vi "SCA-RT_old_new.vi"() -> ()   [LabVIEW 2016]
uses:
  <vilib>/Platform/TimedLoop/XDataNode/wakeup.ctl
  <vilib>/Platform/TimedLoop/XDataNode/XDNodeRunTimeDep.lvlib
  <vilib>/Platform/TimedLoop/XDataNode/nitl_modes.ctl
  <vilib>/Platform/TimedLoop/XDataNode/timing_clust.ctl
  <vilib>/Platform/TimedLoop/XDataNode/XDataNode.xnode
  <vilib>/Motion/BlockNode/FB.NIMotion.xnode
  <vilib>/Platform/TimedLoop/XDataNode/loadnilvce.vi
  controls/state control sample changer.ctl
  <vilib>/Instr/_visa.llb/VISA Configure Serial Port (Instr).vi
  <vilib>/Analysis/NI_AALBase.lvlib
  <vilib>/Analysis/baseanly.llb/Mean (DBL).vi
  controls/SCA states.ctl
  controls/Encoder bit cluster.ctl
  control vi/controls/Gate Valve Readback.ctl
  controls/Horizontal Rod states.ctl
  controls/Vertical Rod states.ctl
  <vilib>/NI_Real-Time Target Support.lvlib
  <vilib>/Motion/Express/_s/nimc.fb.straightLineMove.startStraightLineMove.axis.modeRelative.0.vi
  controls/SCA broadcast status.ctl
  controls/GP307 cluster.ctl
panel:
  out "Timeouts":T1
  out "Encoder loop error":errorcluster
  out "Convectron readback loop error":errorcluster
  out "HV Control loop error":errorcluster
  out "Rotate Wheel error":errorcluster
  out "Ion Source Vac Cluster":T2
  out "Bellows Vac Cluster":T2
  out "Start Sample Change":bool
  out "SCA-cRIO error":errorcluster
  in  "Rollover Sample":i8=54
  out "Insert Rod Status":T3
  out "Retract Rod Status":T3
  out "Sample Rod status":T4
  out "Wheel GV":T5
  out "Raw bits":bool[](array[boolean])
  out "Converted bits":bool[](array[boolean])
  out "Immersion Lens I read":dbl format="%0.2f"
  out "Immersion Lens V read":dbl format="%0.2f"
  out "SCA next state":T6
  out "Extractor I read":dbl
  out "Extractor V read":dbl
  out "Extractor V set":dbl
  out "Cathode V read":dbl
  out "Cathode I read":dbl
  out "Cathode V set":dbl
  in  "Execute Move":bool
  out "New Move":dbl
  out "Encoder Destination":dbl
  in  "Step Window Radius":i16=2
  out "In Range?":bool
  out "Window Limit 2":u32
  out "Window Limit 1":u32
  out "Encoder position":u16
  out "change sample start end":bool
  out "start sample change":bool
  in  "clear error 3":bool
  in  "clear error 2":bool
  out "set cold cathode on 2":bool
  out "Rotate Wheel":bool
  out "Venting Source":bool
  out "Pumping out Source":bool
  out "insert Retract Rod":bool
  out "retract Retract Rod":bool
  out "Open Wheel GV":bool
  out "Close Wheel GV":bool
  out "insert Insert Rod":bool
  out "retract Insert Rod":bool
  out "insert Sample Rod":bool
  out "retract Sample Rod":bool
  in  "clear error":bool
  out "action":string
  out "Vac Readback Loop error":errorcluster
  out "Sample Wheel Convectron":string
  out "Sample Rod UP sensor":bool
  out "Sample Rod DOWN sensor":bool
  out "done":bool
  out "Insert Rod IN sensor":bool
  out "Insert Rod OUT sensor":bool
  out "Retract Rod IN sensor":bool
  out "Retract Rod OUT sensor":bool
  out "Sensor loop error":errorcluster
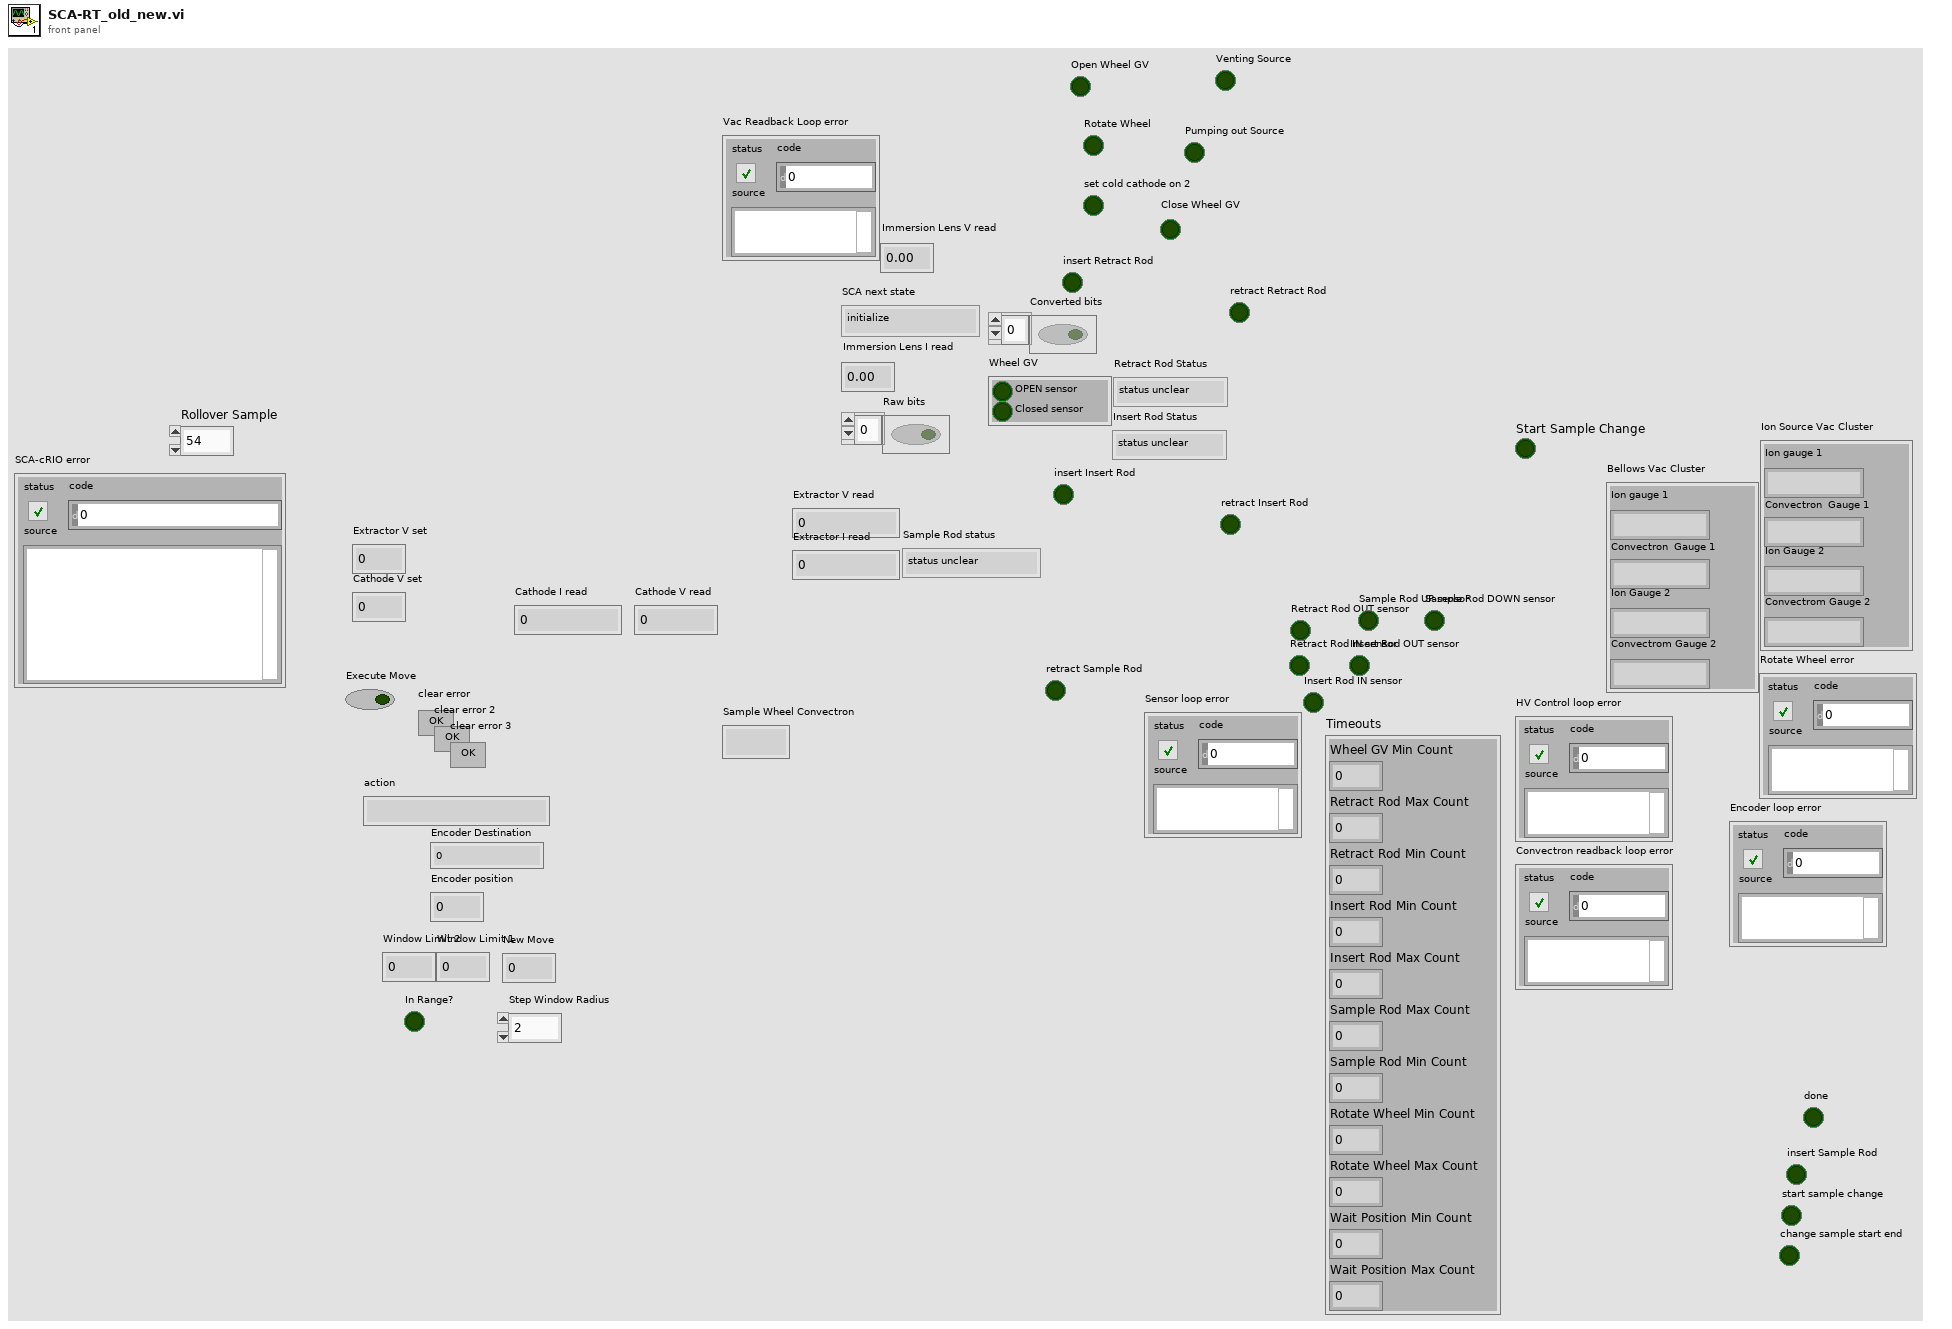
[diagram p1: front panel]
types:
  T1 = cluster{"Wheel GV Min Count":i32, "Retract Rod Max Count":u32, "Retract Rod Min Count":u32, "Insert Rod Min Count":u32, "Insert Rod Max Count":u32, "Sample Rod Max Count":u32, "Sample Rod Min Count":u32, "Rotate Wheel Min Count":u32, "Rotate Wheel Max Count":u32, "Wait Position Min Count":u32, "Wait Position Max Count":u32}
  T2 = typedef "GP307 cluster.ctl" = cluster{"Ion gauge 1":string, "Convectron  Gauge 1 ":string, "Ion Gauge 2":string, "Convectrom Gauge 2":string}
  T3 = typedef "Horizontal Rod states.ctl" = enum16{"status unclear", "rod in", "rod out"}
  T4 = typedef "Vertical Rod states.ctl" = enum16{"status unclear", "rod down", "rod up"}
  T5 = typedef "Gate Valve Readback.ctl" = cluster{"OPEN sensor":bool, "Closed sensor":bool}
  T6 = typedef "SCA states.ctl" = enum16{"initialize", "wait", "change sample start", "change sample", "check position", "rotate wheel", "sample change complete", "sample rod up", "sample rod down", "retract rod in", "retract rod out", "insert rod in", "insert rod out", "wheel GV open", "wheel GV close", "vent source", "pump source", "shutdown"}
  T7 = typedef "SCA broadcast status.ctl" = enum16{"Waiting", "Changing samples", "Sample change complete", "Failure"}
  T8 = typedef "SCA states.ctl" = enum16{"initialize", "wait", "change sample start", "change sample", "check position", "wait position", "rotate wheel", "sample change complete", "sample rod up", "sample rod down", "retract rod in", "retract rod out", "insert rod in", "insert rod out", "wheel GV open", "wheel GV close", "vent source", "pump source"}
  T9 = typedef "GV states.ctl" = enum16{"status unclear", "closed", "open"}
  T10 = typedef "XDNodeRunTimeDep.lvlib/timing_clust.ctl" = cluster{"Expected End [f-1]":u64, "Actual End [f-1]":u64, "Finished Late? [f-1]":bool, "Expected End [i-1]":u64, "Actual End [i-1]":u64, "Finished Late? [i-1]":bool, "Expected Start [i]":u64, "Actual Start [i]":u64, "Expected Start [f]":u64, "Actual Start [f]":u64, "Source Name":string, "Structure Name":string, "Period":i64, "Deadline":i64, "Offset":i64, "Start":i64, "Priority":i32, "Timeout":i32, "Mode":T11, "Wakeup Reason":T12, "Error":errorcluster, "Source Type":string, "Secondary Source Type":string, "Global End Time":u64, "Global Start Time":u64, "Frame Duration":u64, "Iteration Duration":u64, "Assigned CPU":i32, "I/O Scan Engine Mode":u32}
  T11 = typedef "XDNodeRunTimeDep.lvlib/nitl_modes.ctl" = enum32{"No Change", "Process missed periods, maintain original phase", "Discard missed periods, maintain original phase", "Process missed periods, ignore original phase", "Discard missed periods, ignore original phase"}
  T12 = typedef "XDNodeRunTimeDep.lvlib/wakeup.ctl" = enum32{"Normal", "Aborted", "Asynchronous wakeup", "Timing source error", "Timed loop error", "Timeout"}
  T13 = typedef "Encoder bit cluster.ctl" = cluster{"MSB":bool, "13th bit":bool, "12th bit":bool, "11th bit":bool, "10th bit":bool, "9th bit":bool, "8th bit":bool, "7th bit":bool, "6th bit":bool, "5th bit":bool, "4th bit":bool, "3rd bit":bool, "2nd bit":bool, "LSB":bool}
  T14 = typedef "state control sample changer.ctl" = string
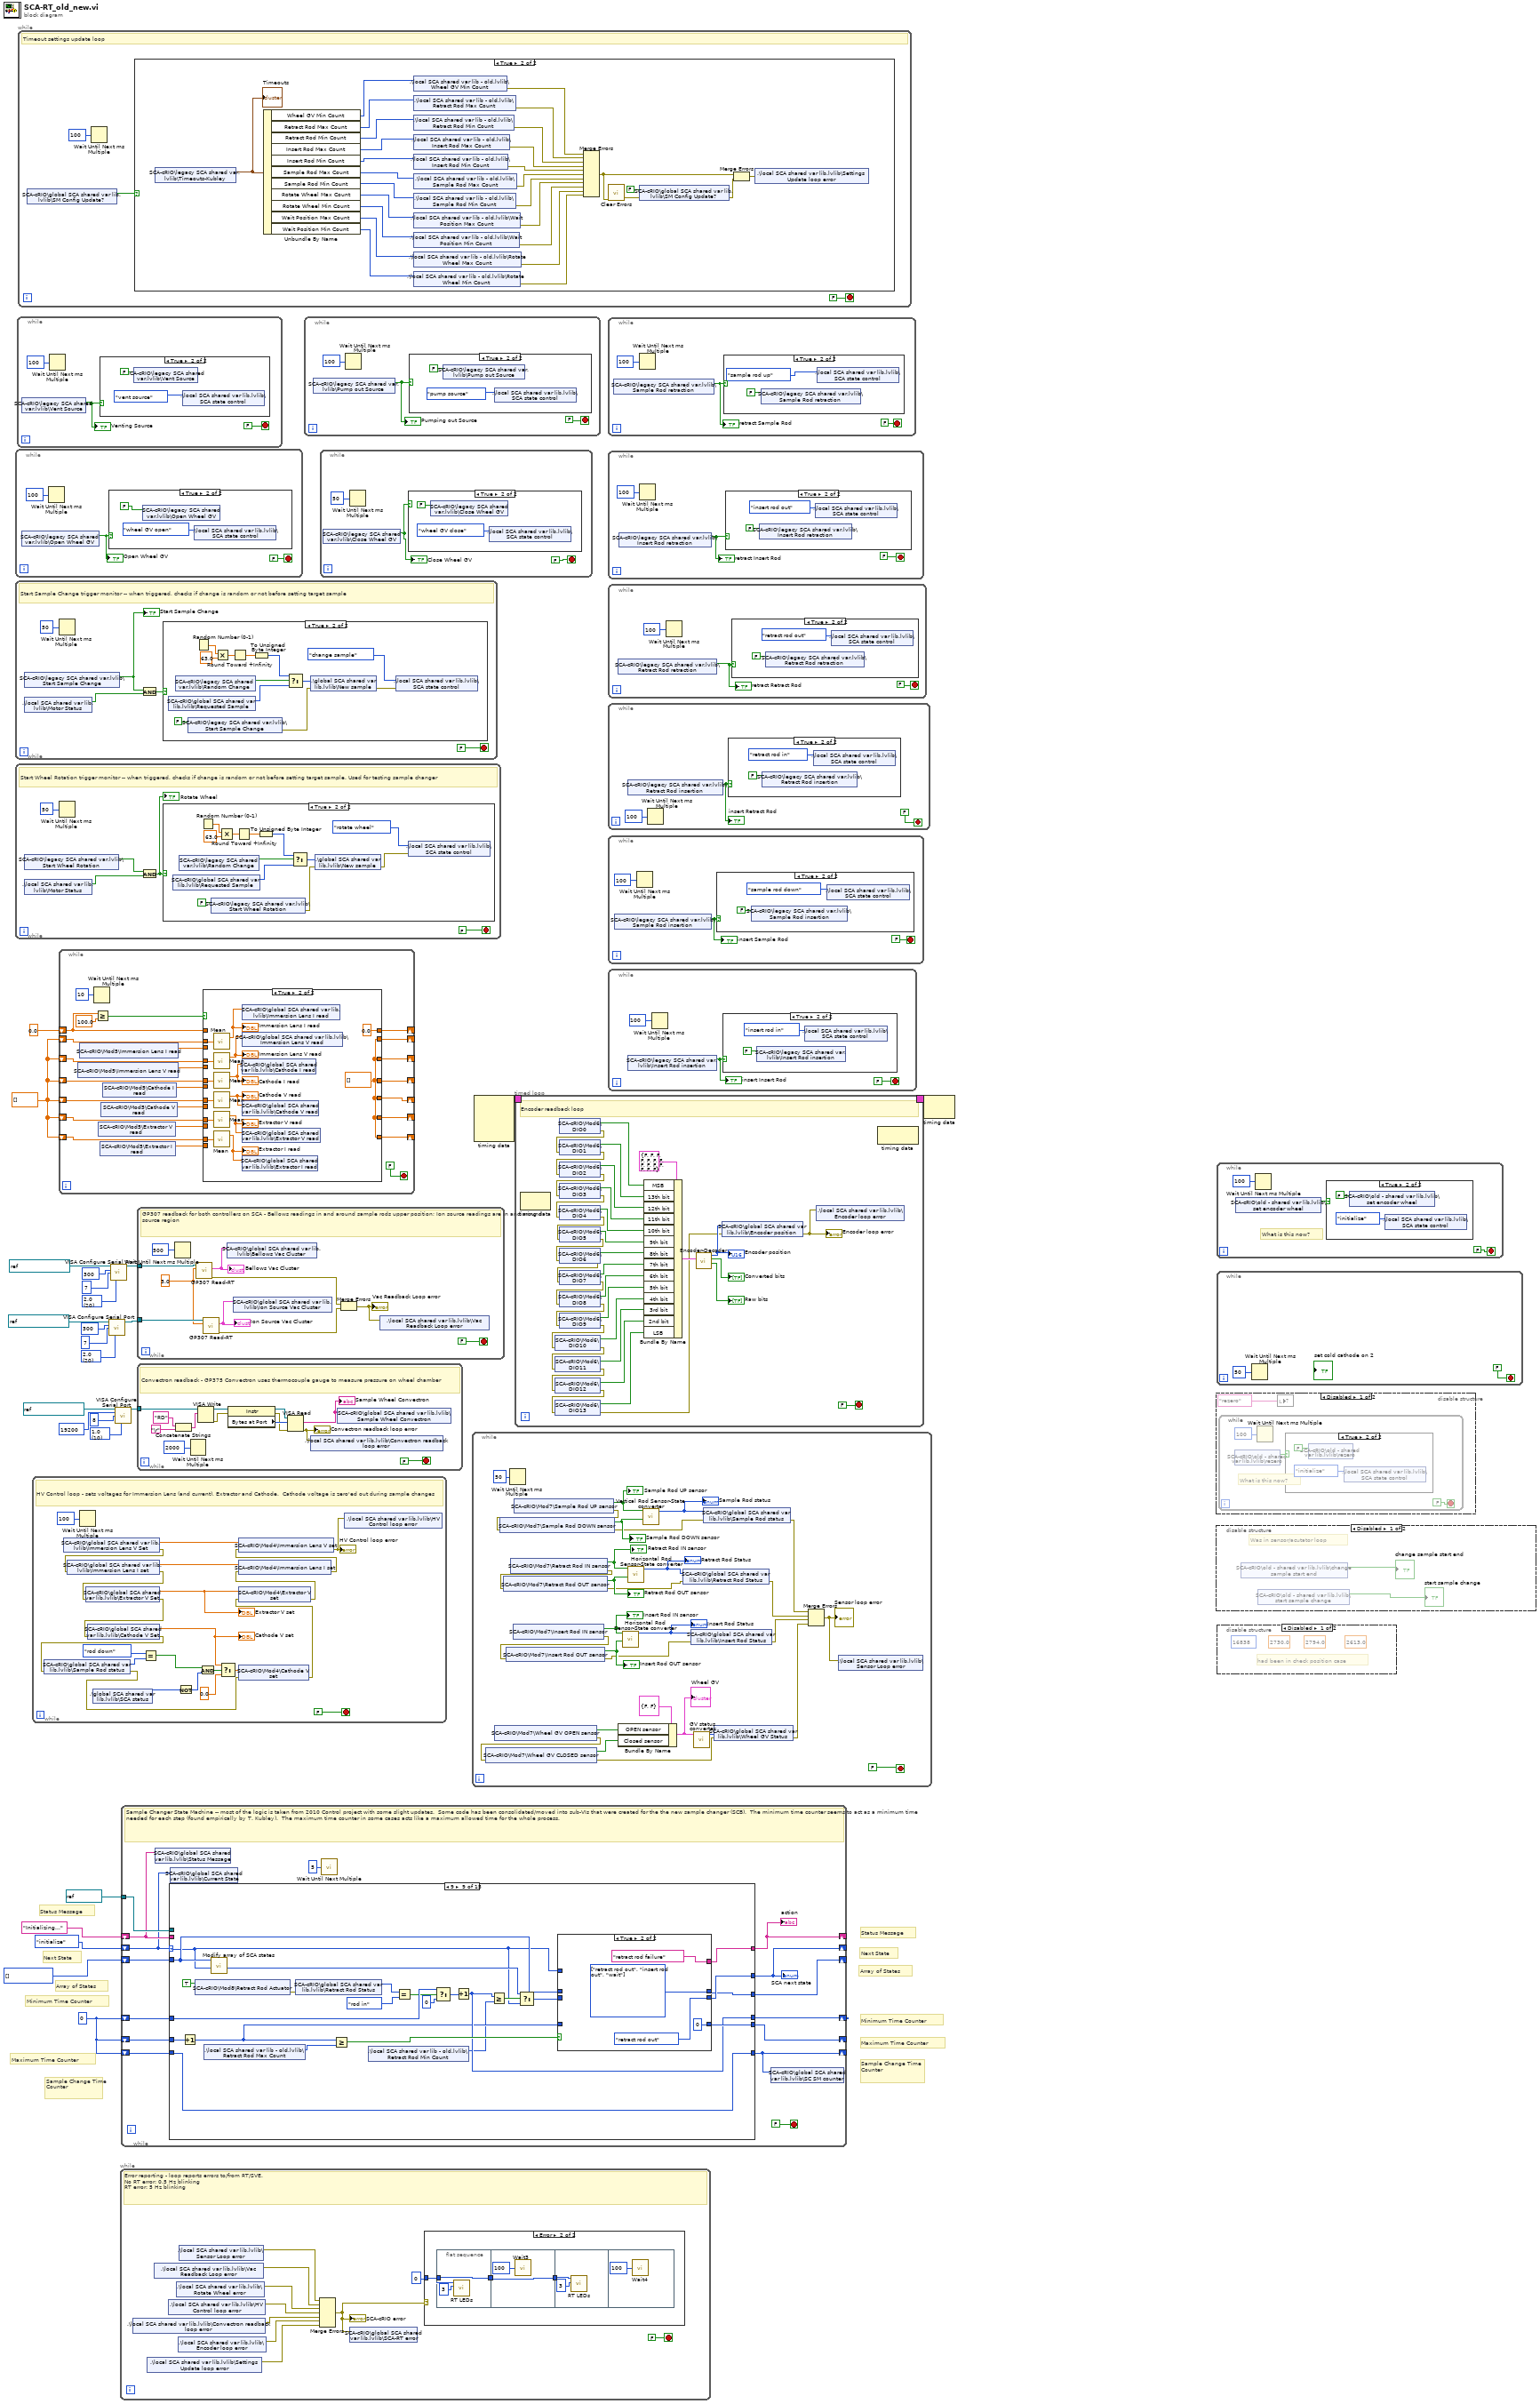
[diagram p0: block diagram]
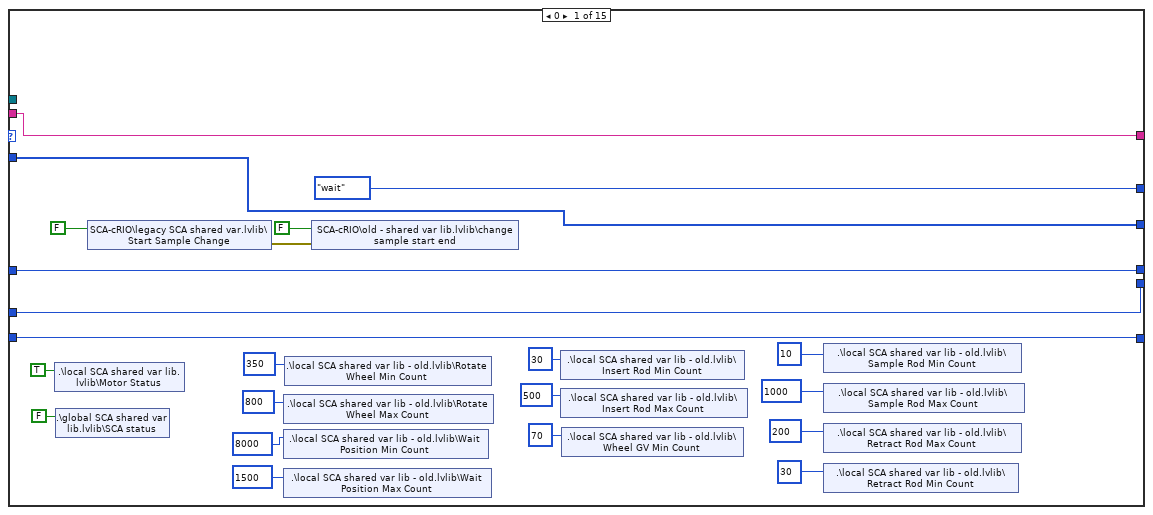
[diagram p5: hidden frame]
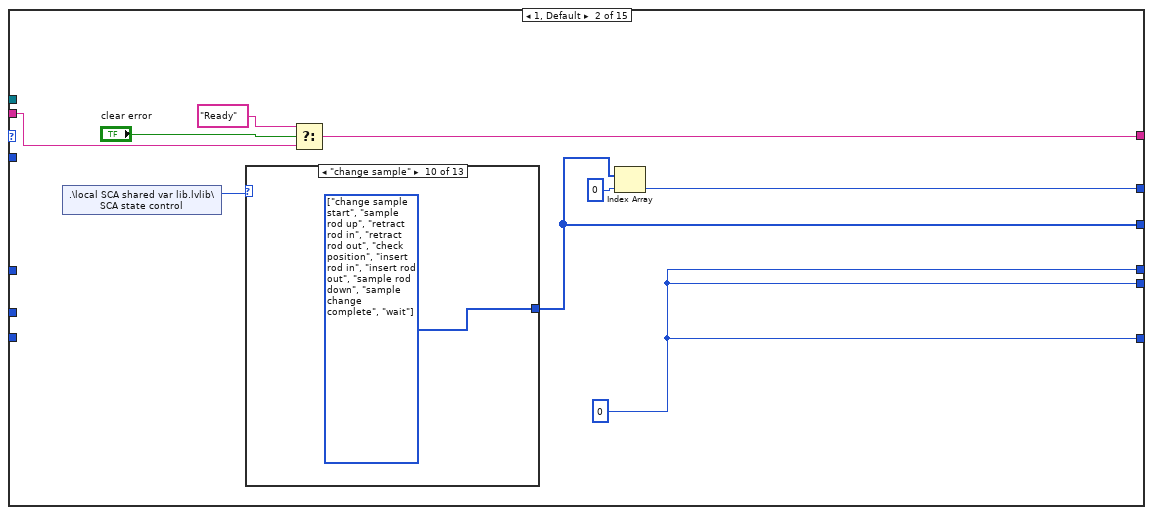
[diagram p6: hidden frame]
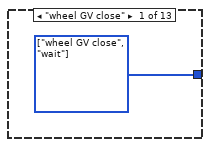
[diagram p7: hidden frame]
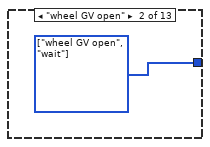
[diagram p8: hidden frame]
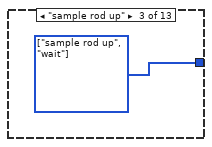
[diagram p9: hidden frame]
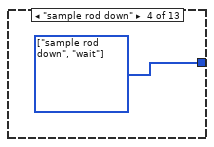
[diagram p10: hidden frame]
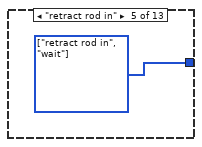
[diagram p11: hidden frame]
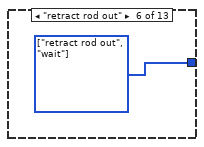
[diagram p12: hidden frame]
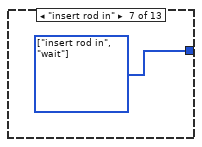
[diagram p13: hidden frame]
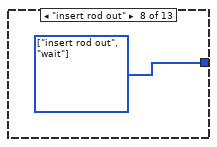
[diagram p14: hidden frame]
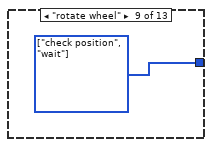
[diagram p15: hidden frame]
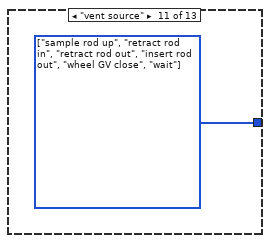
[diagram p16: hidden frame]
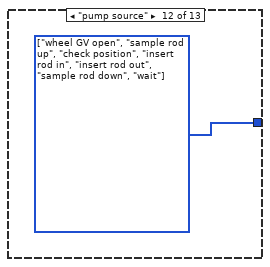
[diagram p17: hidden frame]
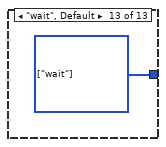
[diagram p18: hidden frame]
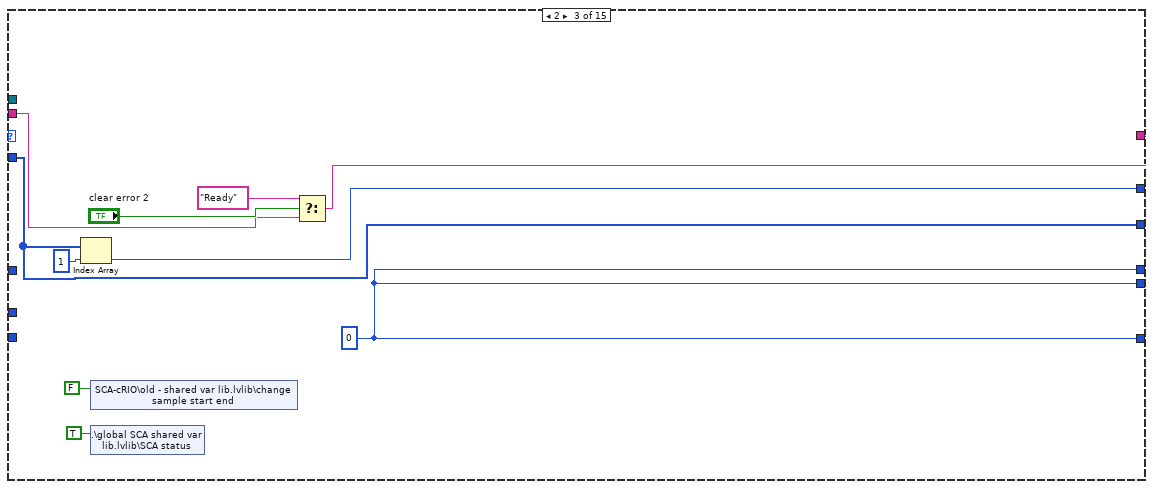
[diagram p19: hidden frame]
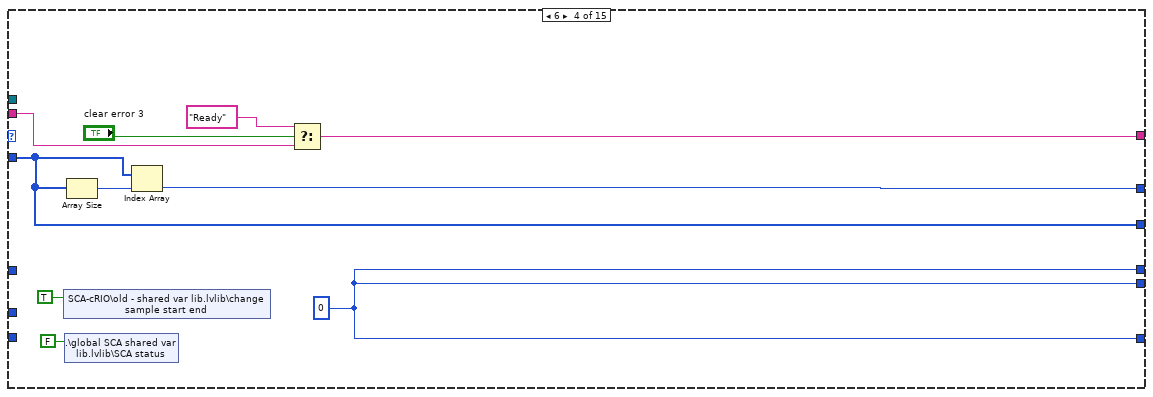
[diagram p20: hidden frame]
diagram:
  w2 = dbl[] []
  w19 = u16 20 items=["1.0"=10, "1.5"=15, "2.0"=20] ("stop bits (10: 1 bit)")
  w23 = u16 10 items=["1.0"=10, "1.5"=15, "2.0"=20] ("stop bits (10: 1 bit)")
  w13 = u16 20 items=["1.0"=10, "1.5"=15, "2.0"=20] ("stop bits (10: 1 bit)")
  w7 = u32 0
  w24 = T6[] [] items=["initialize", "wait", "change sample start", "change sample", "check position", "rotate wheel", "sample change complete", "sample rod up", "sample rod down", "retract rod in", "retract rod out", "insert rod in", "insert rod out", "wheel GV open", "wheel GV close", "vent source", "pump source", "shutdown"]
  # "Status Message"
  # "Array of States"
  # "Next State"
  # "Sample Change Time Counter"
  # "Maximum Time Counter"
  # "Minimum Time Counter"
  # "Status Message"
  # "Array of States"
  # "Next State"
  # "Sample Change Time Counter"
  # "Maximum Time Counter"
  # "Minimum Time Counter"
  n1 = while {
    stop <- FALSE stop-if-true
    n2 = shared-variable "SCA-cRIO\\legacy SCA shared var.lvlib\\Open Wheel GV"() -> (w26:bool)  [unwired: 1 in, 1 out]
    "Open Wheel GV" <- w26
    n3 = Wait Until Next ms Multiple(millisecond multiple=u32 100) -> ()  [unwired: 1 out]
    n4 = case shown="True" w26 {
      frame False {
      }
      frame True {
        n5 = shared-variable "SCA-cRIO\\legacy SCA shared var.lvlib\\Open Wheel GV"(FALSE ("rod up shared")) -> ()  [unwired: 1 in, 1 out]
        n6 = shared-variable ".\\local SCA shared var lib.lvlib\\SCA state control"(SCA_states."wheel GV open" ("SC2 state")) -> ()  [unwired: 1 in, 1 out]
      }
    }
  }
  n7 = while {
    stop <- FALSE stop-if-true
    # "Start Sample Change trigger monitor -- when triggered, checks if change is random or not before setting target sample"
    n8 = shared-variable "SCA-cRIO\\legacy SCA shared var.lvlib\\Start Sample Change"() -> (w32:bool)  [unwired: 1 in, 1 out]
    "Start Sample Change" <- w32
    n9 = shared-variable ".\\local SCA shared var lib.lvlib\\Motor Status"() -> (w30:bool)  [unwired: 1 in, 1 out]
    n10 = Wait Until Next ms Multiple(millisecond multiple=u32 50) -> ()  [unwired: 1 out]
    n11 = And(x=w32, y=w30) -> (x .and. y?=w31:bool)
    n12 = case shown="True" w31 {
      frame False {
      }
      frame True {
        n13 = shared-variable "SCA-cRIO\\global SCA shared var lib.lvlib\\Requested Sample"() -> (w38:u8)  [unwired: 1 in, 1 out]
        n14 = shared-variable "SCA-cRIO\\legacy SCA shared var.lvlib\\Random Change"() -> (w37:bool)  [unwired: 1 in, 1 out]
        n15 = shared-variable "SCA-cRIO\\legacy SCA shared var.lvlib\\Start Sample Change"(FALSE ("rod up shared")) -> (error out=w35:errorcluster)  [unwired: 1 in]
        n16 = Random Number (0-1)() -> (number: 0 to 1=w42:dbl)
        n17 = Multiply(x=w42, y=63.0) -> (x*y=w40:dbl)
        n18 = Round Toward +Infinity(x=w40) -> (ceil(x): smallest int >= x=w43:dbl)
        n19 = To Unsigned Byte Integer(number=w43) -> (unsigned 8bit integer=w44:u8)
        n20 = Select(t=w44, s=w37, f=w38) -> (s? t:f=w39:u8)
        n21 = shared-variable ".\\global SCA shared var lib.lvlib\\New sample"(w39, error in=w35) -> (error out=w36:errorcluster)
        n22 = shared-variable ".\\local SCA shared var lib.lvlib\\SCA state control"(SCA_states."change sample" ("SC2 state"), error in=w36) -> ()  [unwired: 1 out]
      }
    }
  }
  n23 = while {
    stop <- FALSE stop-if-true
    # "Start Wheel Rotation trigger monitor -- when triggered, checks if change is random or not before setting target sample. Used for testing sample changer"
    n24 = shared-variable "SCA-cRIO\\legacy SCA shared var.lvlib\\Start Wheel Rotation"() -> (w49:bool)  [unwired: 1 in, 1 out]
    n25 = shared-variable ".\\local SCA shared var lib.lvlib\\Motor Status"() -> (w48:bool)  [unwired: 1 in, 1 out]
    n26 = Wait Until Next ms Multiple(millisecond multiple=u32 50) -> ()  [unwired: 1 out]
    n27 = And(x=w49, y=w48) -> (x .and. y?=w47:bool)
    "Rotate Wheel" <- w47
    n28 = case shown="True" w47 {
      frame False {
      }
      frame True {
        n29 = shared-variable "SCA-cRIO\\global SCA shared var lib.lvlib\\Requested Sample"() -> (w55:u8)  [unwired: 1 in, 1 out]
        n30 = shared-variable "SCA-cRIO\\legacy SCA shared var.lvlib\\Random Change"() -> (w54:bool)  [unwired: 1 in, 1 out]
        n31 = Random Number (0-1)() -> (number: 0 to 1=w59:dbl)
        n32 = shared-variable "SCA-cRIO\\legacy SCA shared var.lvlib\\Start Wheel Rotation"(FALSE ("rod up shared")) -> (error out=w52:errorcluster)  [unwired: 1 in]
        n33 = Multiply(x=w59, y=63.0) -> (x*y=w57:dbl)
        n34 = Round Toward +Infinity(x=w57) -> (ceil(x): smallest int >= x=w60:dbl)
        n35 = To Unsigned Byte Integer(number=w60) -> (unsigned 8bit integer=w61:u8)
        n36 = Select(t=w61, s=w54, f=w55) -> (s? t:f=w56:u8)
        n37 = shared-variable ".\\global SCA shared var lib.lvlib\\New sample"(w56, error in=w52) -> (error out=w53:errorcluster)
        n38 = shared-variable ".\\local SCA shared var lib.lvlib\\SCA state control"(SCA_states."rotate wheel" ("SC2 state"), error in=w53) -> ()  [unwired: 1 out]
      }
    }
  }
  n39 = while {
    stop <- FALSE stop-if-true
    n40 = shared-variable "SCA-cRIO\\legacy SCA shared var.lvlib\\Vent Source"() -> (w65:bool)  [unwired: 1 in, 1 out]
    "Venting Source" <- w65
    n41 = Wait Until Next ms Multiple(millisecond multiple=u32 100) -> ()  [unwired: 1 out]
    n42 = case shown="True" w65 {
      frame False {
      }
      frame True {
        n43 = shared-variable "SCA-cRIO\\legacy SCA shared var.lvlib\\Vent Source"(FALSE ("rod up shared")) -> ()  [unwired: 1 in, 1 out]
        n44 = shared-variable ".\\local SCA shared var lib.lvlib\\SCA state control"(SCA_states."vent source" ("SCA state control")) -> ()  [unwired: 1 in, 1 out]
      }
    }
  }
  n45 = while {
    stop <- FALSE stop-if-true
    # "Timeout settings update loop"
    n46 = shared-variable "SCA-cRIO\\global SCA shared var lib.lvlib\\SM Config Update?"() -> (w71:bool)  [unwired: 1 in, 1 out]
    n47 = Wait Until Next ms Multiple(millisecond multiple=u32 100) -> ()  [unwired: 1 out]
    n48 = case shown="True" w71 {
      frame False {
      }
      frame True {
        n49 = shared-variable "SCA-cRIO\\legacy SCA shared var.lvlib\\Timeouts-Kubley"() -> (w98:T1)  [unwired: 1 in, 1 out]
        "Timeouts" <- w98
        n50 = Unbundle By Name(w98) -> ("Wheel GV Min Count"=w97:i32, "Retract Rod Max Count"=w96:u32, "Retract Rod Min Count"=w95:u32, "Insert Rod Max Count"=w94:u32, "Insert Rod Min Count"=w93:u32, "Sample Rod Max Count"=w92:u32, "Sample Rod Min Count"=w91:u32, "Rotate Wheel Max Count"=w90:u32, "Rotate Wheel Min Count"=w89:u32, "Wait Position Max Count"=w88:u32, "Wait Position Min Count"=w87:u32)
        n51 = shared-variable ".\\local SCA shared var lib - old.lvlib\\Wheel GV Min Count"(w97) -> (error out=w86:errorcluster)  [unwired: 1 in]
        n52 = shared-variable ".\\local SCA shared var lib - old.lvlib\\Retract Rod Max Count"(w96) -> (error out=w85:errorcluster)  [unwired: 1 in]
        n53 = shared-variable ".\\local SCA shared var lib - old.lvlib\\Retract Rod Min Count"(w95) -> (error out=w84:errorcluster)  [unwired: 1 in]
        n54 = shared-variable ".\\local SCA shared var lib - old.lvlib\\Insert Rod Max Count"(w94) -> (error out=w83:errorcluster)  [unwired: 1 in]
        n55 = shared-variable ".\\local SCA shared var lib - old.lvlib\\Insert Rod Min Count"(w93) -> (error out=w82:errorcluster)  [unwired: 1 in]
        n56 = shared-variable ".\\local SCA shared var lib - old.lvlib\\Sample Rod Max Count"(w92) -> (error out=w81:errorcluster)  [unwired: 1 in]
        n57 = shared-variable ".\\local SCA shared var lib - old.lvlib\\Sample Rod Min Count"(w91) -> (error out=w80:errorcluster)  [unwired: 1 in]
        n58 = shared-variable ".\\local SCA shared var lib - old.lvlib\\Wait Position Max Count"(w90) -> (error out=w79:errorcluster)  [unwired: 1 in]
        n59 = shared-variable ".\\local SCA shared var lib - old.lvlib\\Wait Position Min Count"(w89) -> (error out=w78:errorcluster)  [unwired: 1 in]
        n60 = shared-variable ".\\local SCA shared var lib - old.lvlib\\Rotate Wheel Max Count"(w88) -> (error out=w77:errorcluster)  [unwired: 1 in]
        n61 = shared-variable ".\\local SCA shared var lib - old.lvlib\\Rotate Wheel Min Count"(w87) -> (error out=w76:errorcluster)  [unwired: 1 in]
        n62 = Merge Errors(w86, w85, w84, w83, w82, w81, w80, w79, w78, w77, w76) -> (w74:errorcluster)
        n63 = call <vilib>:"Clear Errors.vi"("error in (no error)"=w74) -> ("error out"=w75:errorcluster)  [unwired: 5 in, 1 out]
        n64 = shared-variable "SCA-cRIO\\global SCA shared var lib.lvlib\\SM Config Update?"(FALSE ("SM Config Update?"), error in=w75) -> (error out=w73:errorcluster)
        n65 = Merge Errors(w74, w73) -> (w72:errorcluster)
        n66 = shared-variable ".\\local SCA shared var lib.lvlib\\Settings Update loop error"(w72) -> ()  [unwired: 1 in, 1 out]
      }
    }
  }
  n67 = while {
    stop <- FALSE stop-if-true
    # "HV Control loop - sets voltages for Immersion Lens (and current), Extractor and Cathode.  Cathode voltage is zero'ed out during sample changes"
    n68 = shared-variable "SCA-cRIO\\global SCA shared var lib.lvlib\\Immersion Lens V Set"() -> (w114:dbl, error out=w112:errorcluster)  [unwired: 1 in]
    n69 = shared-variable "SCA-cRIO\\global SCA shared var lib.lvlib\\Immersion Lens I set"(error in=w112) -> (w113:dbl, error out=w111:errorcluster)
    n70 = Wait Until Next ms Multiple(millisecond multiple=u32 100) -> ()  [unwired: 1 out]
    n71 = shared-variable "SCA-cRIO\\global SCA shared var lib.lvlib\\Extractor V Set"(error in=w111) -> (w120:dbl, error out=w110:errorcluster)
    "Extractor V set" <- w120
    n72 = shared-variable "SCA-cRIO\\global SCA shared var lib.lvlib\\Cathode V Set"(error in=w110) -> (w117:dbl, error out=w109:errorcluster)
    "Cathode V set" <- w117
    n73 = shared-variable "SCA-cRIO\\global SCA shared var lib.lvlib\\Sample Rod status"(error in=w109) -> (w103:T4, error out=w101:errorcluster)
    n74 = shared-variable ".\\global SCA shared var lib.lvlib\\SCA status"() -> (w119:T7)  [unwired: 1 in, 1 out]
    n75 = Equal?(x=Vertical_Rod_states."rod down", y=w103) -> (x = y?=w104:bool)
    n76 = Not(x=w119) -> (.not. x?=w100:u16)
    n77 = And(x=w104, y=w100) -> (x .and. y?=w118:bool)
    n78 = Select(t=w117, s=w118, f=0.0) -> (s? t:f=w115:dbl)
    n79 = shared-variable "SCA-cRIO\\Mod4\\Cathode V set"(w115, error in=w101) -> (error out=w106:errorcluster)
    n80 = shared-variable "SCA-cRIO\\Mod4\\Extractor V set"(w120, error in=w106) -> (error out=w107:errorcluster)
    n81 = shared-variable "SCA-cRIO\\Mod4\\Immersion Lens I set"(w113, error in=w107) -> (error out=w108:errorcluster)
    n82 = shared-variable "SCA-cRIO\\Mod4\\Immersion Lens V set"(w114, error in=w108) -> (error out=w105:errorcluster)
    "HV Control loop error" <- w105
    n83 = shared-variable ".\\local SCA shared var lib.lvlib\\HV Control loop error"(w105) -> ()  [unwired: 1 in, 1 out]
  }
  n84 = while {
    shift-right: [w139] -> _
    shift-left: 0.0 ("AI1") -> [w142]
    shift-right: [w137] -> _
    shift-left: w2 -> [w136]
    shift-right: [w138] -> _
    shift-left: w2 -> [w135]
    shift-right: [w133] -> _
    shift-left: w2 -> [w132]
    shift-right: [w130] -> _
    shift-left: w2 -> [w129]
    shift-right: [w124] -> _
    shift-left: w2 -> [w127]
    shift-right: [w123] -> _
    shift-left: w2 -> [w128]
    stop <- FALSE stop-if-true
    n85 = shared-variable "SCA-cRIO\\Mod5\\Immersion Lens V read"() -> (w125:dbl)  [unwired: 1 in, 1 out]
    n86 = shared-variable "SCA-cRIO\\Mod5\\Immersion Lens I read"() -> (w126:dbl)  [unwired: 1 in, 1 out]
    n87 = Wait Until Next ms Multiple(millisecond multiple=u32 10) -> ()  [unwired: 1 out]
    n88 = Greater Or Equal?(x=w142, y=100.0) -> (x >= y?=w140:bool)
    n89 = shared-variable "SCA-cRIO\\Mod5\\Extractor V read"() -> (w134:dbl)  [unwired: 1 in, 1 out]
    n90 = shared-variable "SCA-cRIO\\Mod5\\Extractor I read"() -> (w131:dbl)  [unwired: 1 in, 1 out]
    n91 = shared-variable "SCA-cRIO\\Mod5\\Cathode V read"() -> (w144:dbl)  [unwired: 1 in, 1 out]
    n92 = shared-variable "SCA-cRIO\\Mod5\\Cathode I read"() -> (w143:dbl)  [unwired: 1 in, 1 out]
    n93 = case shown="True" w140 {
      tunnel: w144 -> [w162 _]
      tunnel: w143 -> [w163 _]
      tunnel: w142 -> [w166 _]
      tunnel: [w165 0.0 ("AI1")] -> w139
      tunnel: [w164 w170] -> w138
      tunnel: [w161 w170] -> w137
      tunnel: w136 -> [w160 w178]
      tunnel: w135 -> [w159 w179]
      tunnel: w134 -> [w158 _]
      tunnel: [w157 w170] -> w133
      tunnel: w132 -> [w156 w177]
      tunnel: w131 -> [w155 _]
      tunnel: [w154 w170] -> w130
      tunnel: w129 -> [w153 w176]
      tunnel: w128 -> [w152 w169]
      tunnel: w127 -> [w151 w168]
      tunnel: w126 -> [w150 _]
      tunnel: w125 -> [w149 _]
      tunnel: [w148 w170] -> w124
      tunnel: [w147 w170] -> w123
      frame False {
        n94 = Build Array (concatenate)(w150, w151) -> (w148:dbl[])
        n95 = Build Array (concatenate)(w149, w152) -> (w147:dbl[])
        n96 = Build Array (concatenate)(w163, w159) -> (w164:dbl[])
        n97 = Build Array (concatenate)(w162, w160) -> (w161:dbl[])
        n98 = Build Array (concatenate)(w158, w156) -> (w157:dbl[])
        n99 = Build Array (concatenate)(w155, w153) -> (w154:dbl[])
        n100 = Increment(x=w166) -> (x+1=w165:dbl)
      }
      frame True {
        w170 = dbl[] []
        n101 = call-poly <vilib>:"Mean.vi"("X"=w168) -> ("mean"=w167:dbl)  [unwired: 1 out]
        "Immersion Lens I read" <- w167
        n102 = call-poly <vilib>:"Mean.vi"("X"=w169) -> ("mean"=w171:dbl)  [unwired: 1 out]
        "Immersion Lens V read" <- w171
        n103 = call-poly <vilib>:"Mean.vi"("X"=w179) -> ("mean"=w175:dbl)  [unwired: 1 out]
        "Cathode I read" <- w175
        n104 = call-poly <vilib>:"Mean.vi"("X"=w178) -> ("mean"=w174:dbl)  [unwired: 1 out]
        "Cathode V read" <- w174
        n105 = call-poly <vilib>:"Mean.vi"("X"=w177) -> ("mean"=w173:dbl)  [unwired: 1 out]
        "Extractor V read" <- w173
        n106 = call-poly <vilib>:"Mean.vi"("X"=w176) -> ("mean"=w172:dbl)  [unwired: 1 out]
        "Extractor I read" <- w172
        n107 = shared-variable "SCA-cRIO\\global SCA shared var lib.lvlib\\Immersion Lens I read"(w167) -> ()  [unwired: 1 in, 1 out]
        n108 = shared-variable "SCA-cRIO\\global SCA shared var lib.lvlib\\Immersion Lens V read"(w171) -> ()  [unwired: 1 in, 1 out]
        n109 = shared-variable "SCA-cRIO\\global SCA shared var lib.lvlib\\Cathode I read"(w175) -> ()  [unwired: 1 in, 1 out]
        n110 = shared-variable "SCA-cRIO\\global SCA shared var lib.lvlib\\Cathode V read"(w174) -> ()  [unwired: 1 in, 1 out]
        n111 = shared-variable "SCA-cRIO\\global SCA shared var lib.lvlib\\Extractor V read"(w173) -> ()  [unwired: 1 in, 1 out]
        n112 = shared-variable "SCA-cRIO\\global SCA shared var lib.lvlib\\Extractor I read"(w172) -> ()  [unwired: 1 in, 1 out]
      }
    }
  }
  n113 = call-poly "VISA Configure Serial Port"("VISA resource name"=refnum<visa-resource-name> "ASRL6::INSTR", "baud rate (9600)"=u32 300, "data bits (8)"=u16 7, "stop bits (10: 1 bit)"=w13) -> ("VISA resource name out"=w14:refnum<visa-resource-name>)  [unwired: 10 in, 1 out]
  n114 = call-poly "VISA Configure Serial Port"("VISA resource name"=refnum<visa-resource-name> "ASRL8::INSTR", "baud rate (9600)"=u32 300, "data bits (8)"=u16 7, "stop bits (10: 1 bit)"=w19) -> ("VISA resource name out"=w20:refnum<visa-resource-name>)  [unwired: 10 in, 1 out]
  n115 = call-poly "VISA Configure Serial Port"("VISA resource name"=refnum<visa-resource-name> "ASRL7::INSTR", "baud rate (9600)"=u32 19200, "data bits (8)"=u16 8, "stop bits (10: 1 bit)"=w23) -> ("VISA resource name out"=w9:refnum<visa-resource-name>)  [unwired: 10 in, 1 out]
  n116 = while {
    stop <- FALSE stop-if-true
    # "Error reporting - loop reports errors to/from RT/SVE. \nNo RT error: 0.5 Hz blinking\nRT error: 5 Hz blinking"
    n117 = shared-variable ".\\local SCA shared var lib.lvlib\\Convectron readback loop error"() -> (w183:errorcluster)  [unwired: 1 in, 1 out]
    n118 = shared-variable ".\\local SCA shared var lib.lvlib\\Settings Update loop error"() -> (w181:errorcluster)  [unwired: 1 in, 1 out]
    n119 = shared-variable ".\\local SCA shared var lib.lvlib\\Vac Readback Loop error"() -> (w188:errorcluster)  [unwired: 1 in, 1 out]
    n120 = shared-variable ".\\local SCA shared var lib.lvlib\\HV Control loop error"() -> (w184:errorcluster)  [unwired: 1 in, 1 out]
    n121 = shared-variable ".\\local SCA shared var lib.lvlib\\Rotate Wheel error"() -> (w185:errorcluster)  [unwired: 1 in, 1 out]
    n122 = shared-variable ".\\local SCA shared var lib.lvlib\\Encoder loop error"() -> (w182:errorcluster)  [unwired: 1 in, 1 out]
    n123 = shared-variable ".\\local SCA shared var lib.lvlib\\Sensor Loop error"() -> (w189:errorcluster)  [unwired: 1 in, 1 out]
    n124 = Merge Errors(w189, w188, w185, w184, w183, w182, w181) -> (w187:errorcluster)
    "SCA-cRIO error" <- w187
    n125 = shared-variable "SCA-cRIO\\global SCA shared var lib.lvlib\\SCA-RT error"(w187) -> ()  [unwired: 1 in, 1 out]
    n126 = case shown="Error" w187 {
      tunnel: 0 -> [w193 w201]
      frame No Error {
        n127 = flat-sequence {
          tunnel: w193 -> [w194]
          tunnel: [w194] -> w191
          tunnel: [w196] -> w192
          tunnel: w191 -> [w196]
          tunnel: w192 -> [w198]
          frame #0 {
            n128 = call <vilib>:"RT LEDs.vi"("State"=3, "LED Num"=w194) -> ()  [unwired: 4 in, 2 out]
          }
          frame #1 {
            n129 = call "Wait"("Count(mSec)"=u16 1000) -> ()  [unwired: 1 out]
          }
          frame #2 {
            n130 = call <vilib>:"RT LEDs.vi"("State"=3, "LED Num"=w198) -> ()  [unwired: 4 in, 2 out]
          }
          frame #3 {
            n131 = call "Wait2"("Count(mSec)"=u16 1000) -> ()  [unwired: 1 out]
          }
        }
      }
      frame Error {
        n132 = flat-sequence {
          tunnel: [w204] -> w203
          tunnel: w201 -> [w204]
          tunnel: w203 -> [w206]
          tunnel: [w206] -> w202
          tunnel: w202 -> [w208]
          frame #0 {
            n133 = call <vilib>:"RT LEDs.vi"("State"=3, "LED Num"=w204) -> ()  [unwired: 4 in, 2 out]
          }
          frame #1 {
            n134 = call "Wait3"("Count(mSec)"=u16 100) -> ()  [unwired: 1 out]
          }
          frame #2 {
            n135 = call <vilib>:"RT LEDs.vi"("State"=3, "LED Num"=w208) -> ()  [unwired: 4 in, 2 out]
          }
          frame #3 {
            n136 = call "Wait4"("Count(mSec)"=u16 100) -> ()  [unwired: 1 out]
          }
        }
      }
    }
  }
  n137 = while {
    shift-right: [w223] -> _
    shift-left: SCA_states."initialize" ("SC2 state") -> [w213]
    shift-right: [w212] -> _
    shift-left: w24 -> [w222]
    shift-right: [w220] -> _
    shift-left: w7 -> [w221]
    shift-right: [w219] -> _
    shift-left: "Initializing..." -> [w214]
    shift-right: [w217] -> _
    shift-left: w7 -> [w218]
    shift-right: [w215] -> _
    shift-left: w7 -> [w216]
    tunnel: refnum<k21> "Axis 1" ("resource") -> [w224]
    stop <- FALSE ("stop 2") stop-if-true
    # "Sample Changer State Machine -- most of the logic is taken from 2010 Control project with some slight updates.  Some code has been consolidated/moved into sub-VIs that were created for the the new sample changer (SCB).  The minimum time counter seems to act as a minimum time needed for each step (found empirically by T. Kubley).  The maximum time counter in some cases acts like a maximum allowed time for the whole process."
    n138 = shared-variable "SCA-cRIO\\global SCA shared var lib.lvlib\\Status Message"(w214) -> ()  [unwired: 1 in, 1 out]
    n139 = case shown="9" w213 {
      selector: w213 -> [_ _ _ _ w298 w316 w339 w373 w407 w441 w475 w509 w545 w600 w630]
      tunnel: w224 -> [_ _ _ _ _ _ _ _ _ _ _ _ w560 _ _]
      tunnel: [SCA_states."wait" ("SC2 state") w249 w279 w289 w303 w322 w347 w381 w415 w449 w483 w517 w554 w601 w640] -> w223
      tunnel: w222 -> [w239 _ w271 w281 w299 w317 w340 w374 w408 w442 w476 w510 w546 w599 w629]
      tunnel: w221 -> [w242 _ _ _ w306 w325 w353 w387 w421 w455 w489 w523 w558 w611 w635]
      tunnel: [w242 w252 w274 w284 w305 w324 w333 w367 w402 w436 w470 w504 w541 w612 w635] -> w220
      tunnel: [w239 w250 w271 w281 w299 w317 w342 w376 w410 w444 w478 w512 w555 w608 w629] -> w212
      tunnel: w214 -> [w240 w255 w277 w287 _ _ _ _ _ _ _ _ _ _ _]
      tunnel: [w240 w254 w276 w286 w302 w321 w349 w383 w417 w451 w485 w519 w553 w607 w639] -> w219
      tunnel: w218 -> [w243 _ _ _ w304 w323 w346 w380 w414 w448 w482 w516 w556 w609 _]
      tunnel: [w243 w252 w274 w284 w291 w320 w344 w378 w412 w446 w480 w514 w549 w603 u32 0 ("t")] -> w217
      tunnel: w216 -> [w244 _ _ _ w301 w319 w343 w377 w411 w445 w479 w513 w540 w596 w638]
      tunnel: [w244 w252 w274 w284 w301 w319 w343 w377 w411 w445 w479 w513 w540 w596 w638] -> w215
      frame 0 {
        n140 = shared-variable ".\\local SCA shared var lib.lvlib\\Motor Status"(TRUE ("Motor Status")) -> ()  [unwired: 1 in, 1 out]
        n141 = shared-variable ".\\global SCA shared var lib.lvlib\\SCA status"(FALSE ("Changing Sample")) -> ()  [unwired: 1 in, 1 out]
        n142 = shared-variable "SCA-cRIO\\legacy SCA shared var.lvlib\\Start Sample Change"(FALSE ("start sample change")) -> (error out=w247:errorcluster)  [unwired: 1 in]
        n143 = shared-variable ".\\local SCA shared var lib - old.lvlib\\Rotate Wheel Max Count"(u32 800 ("Rotate Wheel Max Count")) -> ()  [unwired: 1 in, 1 out]
        n144 = shared-variable ".\\local SCA shared var lib - old.lvlib\\Wait Position Min Count"(u32 8000 ("y")) -> ()  [unwired: 1 in, 1 out]
        n145 = shared-variable ".\\local SCA shared var lib - old.lvlib\\Wait Position Max Count"(u32 1500 ("y")) -> ()  [unwired: 1 in, 1 out]
        n146 = shared-variable ".\\local SCA shared var lib - old.lvlib\\Rotate Wheel Min Count"(u32 350 ("Rotate Wheel Min Count")) -> ()  [unwired: 1 in, 1 out]
        n147 = shared-variable "SCA-cRIO\\old - shared var lib.lvlib\\change sample start end"(FALSE ("change sample start end"), error in=w247) -> ()  [unwired: 1 out]
        n148 = shared-variable ".\\local SCA shared var lib - old.lvlib\\Insert Rod Min Count"(u32 30 ("y")) -> ()  [unwired: 1 in, 1 out]
        n149 = shared-variable ".\\local SCA shared var lib - old.lvlib\\Insert Rod Max Count"(u32 500 ("y")) -> ()  [unwired: 1 in, 1 out]
        n150 = shared-variable ".\\local SCA shared var lib - old.lvlib\\Wheel GV Min Count"(70 ("Wheel GV Min Time")) -> ()  [unwired: 1 in, 1 out]
        n151 = shared-variable ".\\local SCA shared var lib - old.lvlib\\Sample Rod Min Count"(u32 10 ("y")) -> ()  [unwired: 1 in, 1 out]
        n152 = shared-variable ".\\local SCA shared var lib - old.lvlib\\Sample Rod Max Count"(u32 1000 ("y")) -> ()  [unwired: 1 in, 1 out]
        n153 = shared-variable ".\\local SCA shared var lib - old.lvlib\\Retract Rod Max Count"(u32 200 ("y")) -> ()  [unwired: 1 in, 1 out]
        n154 = shared-variable ".\\local SCA shared var lib - old.lvlib\\Retract Rod Min Count"(u32 30 ("y")) -> ()  [unwired: 1 in, 1 out]
      }
      frame 1, Default {
        w252 = u32 0
        n155 = shared-variable ".\\local SCA shared var lib.lvlib\\SCA state control"() -> (w248:T6)  [unwired: 1 in, 1 out]
        n156 = case shown="\"change sample\"" w248 {
          tunnel: [w257 w258 w259 w260 w261 w262 w263 w264 w265 w266 w267 w268 w269] -> w250
          frame "wheel GV close" {
            w257 = T6[] [enum."wheel GV close", enum."wait"] items=["initialize", "wait", "change sample start", "change sample", "check position", "rotate wheel", "sample change complete", "sample rod up", "sample rod down", "retract rod in", "retract rod out", "insert rod in", "insert rod out", "wheel GV open", "wheel GV close", "vent source", "pump source", "shutdown"]
          }
          frame "wheel GV open" {
            w258 = T6[] [enum."wheel GV open", enum."wait"] items=["initialize", "wait", "change sample start", "change sample", "check position", "rotate wheel", "sample change complete", "sample rod up", "sample rod down", "retract rod in", "retract rod out", "insert rod in", "insert rod out", "wheel GV open", "wheel GV close", "vent source", "pump source", "shutdown"]
          }
          frame "sample rod up" {
            w259 = T6[] [enum."sample rod up", enum."wait"] items=["initialize", "wait", "change sample start", "change sample", "check position", "rotate wheel", "sample change complete", "sample rod up", "sample rod down", "retract rod in", "retract rod out", "insert rod in", "insert rod out", "wheel GV open", "wheel GV close", "vent source", "pump source", "shutdown"]
          }
          frame "sample rod down" {
            w260 = T6[] [enum."sample rod down", enum."wait"] items=["initialize", "wait", "change sample start", "change sample", "check position", "rotate wheel", "sample change complete", "sample rod up", "sample rod down", "retract rod in", "retract rod out", "insert rod in", "insert rod out", "wheel GV open", "wheel GV close", "vent source", "pump source", "shutdown"]
          }
          frame "retract rod in" {
            w261 = T6[] [enum."retract rod in", enum."wait"] items=["initialize", "wait", "change sample start", "change sample", "check position", "rotate wheel", "sample change complete", "sample rod up", "sample rod down", "retract rod in", "retract rod out", "insert rod in", "insert rod out", "wheel GV open", "wheel GV close", "vent source", "pump source", "shutdown"]
          }
          frame "retract rod out" {
            w262 = T6[] [enum."retract rod out", enum."wait"] items=["initialize", "wait", "change sample start", "change sample", "check position", "rotate wheel", "sample change complete", "sample rod up", "sample rod down", "retract rod in", "retract rod out", "insert rod in", "insert rod out", "wheel GV open", "wheel GV close", "vent source", "pump source", "shutdown"]
          }
          frame "insert rod in" {
            w263 = T6[] [enum."insert rod in", enum."wait"] items=["initialize", "wait", "change sample start", "change sample", "check position", "rotate wheel", "sample change complete", "sample rod up", "sample rod down", "retract rod in", "retract rod out", "insert rod in", "insert rod out", "wheel GV open", "wheel GV close", "vent source", "pump source", "shutdown"]
          }
          frame "insert rod out" {
            w264 = T6[] [enum."insert rod out", enum."wait"] items=["initialize", "wait", "change sample start", "change sample", "check position", "rotate wheel", "sample change complete", "sample rod up", "sample rod down", "retract rod in", "retract rod out", "insert rod in", "insert rod out", "wheel GV open", "wheel GV close", "vent source", "pump source", "shutdown"]
          }
          frame "rotate wheel" {
            w265 = T6[] [enum."check position", enum."wait"] items=["initialize", "wait", "change sample start", "change sample", "check position", "rotate wheel", "sample change complete", "sample rod up", "sample rod down", "retract rod in", "retract rod out", "insert rod in", "insert rod out", "wheel GV open", "wheel GV close", "vent source", "pump source", "shutdown"]
          }
          frame "change sample" {
            w266 = T6[] [enum."change sample start", enum."sample rod up", enum."retract rod in", enum."retract rod out", enum."check position", enum."insert rod in", enum."insert rod out", enum."sample rod down", enum."sample change complete", enum."wait"] items=["initialize", "wait", "change sample start", "change sample", "check position", "rotate wheel", "sample change complete", "sample rod up", "sample rod down", "retract rod in", "retract rod out", "insert rod in", "insert rod out", "wheel GV open", "wheel GV close", "vent source", "pump source", "shutdown"]
          }
          frame "vent source" {
            w267 = T6[] [enum."sample rod up", enum."retract rod in", enum."retract rod out", enum."insert rod out", enum."wheel GV close", enum."wait"] items=["initialize", "wait", "change sample start", "change sample", "check position", "rotate wheel", "sample change complete", "sample rod up", "sample rod down", "retract rod in", "retract rod out", "insert rod in", "insert rod out", "wheel GV open", "wheel GV close", "vent source", "pump source", "shutdown"]
          }
          frame "pump source" {
            w268 = T6[] [enum."wheel GV open", enum."sample rod up", enum."check position", enum."insert rod in", enum."insert rod out", enum."sample rod down", enum."wait"] items=["initialize", "wait", "change sample start", "change sample", "check position", "rotate wheel", "sample change complete", "sample rod up", "sample rod down", "retract rod in", "retract rod out", "insert rod in", "insert rod out", "wheel GV open", "wheel GV close", "vent source", "pump source", "shutdown"]
          }
          frame "wait", Default {
            w269 = T6[] [enum."wait"] items=["initialize", "wait", "change sample start", "change sample", "check position", "rotate wheel", "sample change complete", "sample rod up", "sample rod down", "retract rod in", "retract rod out", "insert rod in", "insert rod out", "wheel GV open", "wheel GV close", "vent source", "pump source", "shutdown"]
          }
        }
        n157 = Select(t="Ready", s="clear error", f=w255) -> (s? t:f=w254:string)
        n158 = Index Array(array=w250, index=0) -> (element=w249:T6)
      }
      frame 2 {
        w274 = u32 0
        n159 = Index Array(array=w271, index=1) -> (element=w279:T6)
        n160 = shared-variable "SCA-cRIO\\old - shared var lib.lvlib\\change sample start end"(FALSE ("change sample start end")) -> ()  [unwired: 1 in, 1 out]
        n161 = shared-variable ".\\global SCA shared var lib.lvlib\\SCA status"(TRUE ("Changing Sample")) -> ()  [unwired: 1 in, 1 out]
        n162 = Select(t="Ready", s="clear error 2", f=w277) -> (s? t:f=w276:string)
      }
      frame 6 {
        w284 = u32 0
        n163 = shared-variable "SCA-cRIO\\old - shared var lib.lvlib\\change sample start end"(TRUE ("change sample start end")) -> ()  [unwired: 1 in, 1 out]
        n164 = shared-variable ".\\global SCA shared var lib.lvlib\\SCA status"(FALSE ("Changing Sample")) -> ()  [unwired: 1 in, 1 out]
        n165 = Array Size(array=w281) -> (size(s)=w282:i32)
        n166 = Index Array(array=w281, index=w282) -> (element=w289:T6)
        n167 = Select(t="Ready", s="clear error 3", f=w287) -> (s? t:f=w286:string)
      }
      frame 13 {
        n168 = call "Modify array of SCA states.vi"("Current State"=w298, "Array of states to process"=w299) -> ("Next State"=w300:T6)  [unwired: 7 in, 1 out]
        n169 = shared-variable "SCA-cRIO\\Mod8\\Wheel GV Actuator"(TRUE ("sc gate valve")) -> (error out=w296:errorcluster)  [unwired: 1 in]
        n170 = shared-variable "SCA-cRIO\\global SCA shared var lib.lvlib\\Wheel GV Status"(error in=w296) -> (w295:enum16{"status unclear", "closed", "open"})  [unwired: 1 out]
        n171 = shared-variable ".\\local SCA shared var lib - old.lvlib\\Wheel GV Min Count"() -> (w290:i32)  [unwired: 1 in, 1 out]
        n172 = Equal?(x=enum16{"status unclear", "closed", "open"}."open", y=w295) -> (x = y?=w293:bool)
        n173 = Select(t=w306, s=w293, f=u32 0) -> (s? t:f=w309:u32)
        n174 = Increment(x=w309) -> (x+1=w305:u32)
        n175 = Greater Or Equal?(x=w305, y=w290) -> (x >= y?=w307:bool)
        n176 = Select(t=w300, s=w307, f=w298) -> (s? t:f=w303:u16)
        n177 = Increment(x=w304) -> (x+1=w291:u32)
        n178 = Format Into String(format string="%s", w298) -> (resulting string=w302:string)  [unwired: 2 in, 1 out]
      }
      frame 14 {
        n179 = call "Modify array of SCA states.vi"("Current State"=w316, "Array of states to process"=w317) -> ("Next State"=w318:T6)  [unwired: 7 in, 1 out]
        n180 = shared-variable "SCA-cRIO\\Mod8\\Wheel GV Actuator"(FALSE ("sc gate valve")) -> (error out=w314:errorcluster)  [unwired: 1 in]
        n181 = shared-variable "SCA-cRIO\\global SCA shared var lib.lvlib\\Wheel GV Status"(error in=w314) -> (w313:enum16{"status unclear", "closed", "open"})  [unwired: 1 out]
        n182 = shared-variable ".\\local SCA shared var lib - old.lvlib\\Wheel GV Min Count"() -> (w329:i32)  [unwired: 1 in, 1 out]
        n183 = Equal?(x=enum16{"status unclear", "closed", "open"}."closed", y=w313) -> (x = y?=w311:bool)
        n184 = Select(t=w325, s=w311, f=u32 0) -> (s? t:f=w328:u32)
        n185 = Increment(x=w328) -> (x+1=w324:u32)
        n186 = Greater Or Equal?(x=w324, y=w329) -> (x >= y?=w326:bool)
        n187 = Select(t=w318, s=w326, f=w316) -> (s? t:f=w322:u16)
        n188 = Increment(x=w323) -> (x+1=w320:u32)
        n189 = Format Into String(format string="%s", w316) -> (resulting string=w321:string)  [unwired: 2 in, 1 out]
      }
      frame 7 {
        n190 = Increment(x=w346) -> (x+1=w332:u32)
        n191 = shared-variable "SCA-cRIO\\Mod8\\Sample Rod Actuator"(FALSE ("Sample Rod Actuator")) -> (error out=w337:errorcluster)  [unwired: 1 in]
        n192 = shared-variable ".\\local SCA shared var lib - old.lvlib\\Sample Rod Max Count"() -> (w331:u32)  [unwired: 1 in, 1 out]
        n193 = call "Modify array of SCA states.vi"("Current State"=w339, "Array of states to process"=w340) -> ("Next State"=w341:T6)  [unwired: 7 in, 1 out]
        n194 = shared-variable "SCA-cRIO\\global SCA shared var lib.lvlib\\Sample Rod status"(error in=w337) -> (w336:T4)  [unwired: 1 out]
        n195 = Greater Or Equal?(x=w332, y=w331) -> (x >= y?=w345:bool)
        n196 = shared-variable ".\\local SCA shared var lib - old.lvlib\\Sample Rod Min Count"() -> (w330:u32)  [unwired: 1 in, 1 out]
        n197 = Equal?(x=w336, y=Vertical_Rod_states."rod up") -> (x = y?=w334:bool)
        n198 = Select(t=w353, s=w334, f=u32 0) -> (s? t:f=w351:u32)
        n199 = Increment(x=w351) -> (x+1=w333:u32)
        n200 = Greater Or Equal?(x=w333, y=w330) -> (x >= y?=w352:bool)
        n201 = Select(t=w341, s=w352, f=w339) -> (s? t:f=w348:u16)
        n202 = case shown="False" w345 {
          tunnel: [w359 u32 0] -> w344
          tunnel: [w357 w360] -> w342
          tunnel: [w358 SCA_states."wait" ("SC2 state")] -> w347
          tunnel: w332 -> [w359 _]
          tunnel: w339 -> [w355 _]
          tunnel: [w354 "sample rod failure"] -> w349
          tunnel: w348 -> [w358 _]
          tunnel: w340 -> [w357 _]
          frame False {
            n203 = Format Into String(format string="%s", w355) -> (resulting string=w354:string)  [unwired: 2 in, 1 out]
          }
          frame True {
            w360 = T6[] [enum."wait", enum."insert rod out", enum."wait"] items=["initialize", "wait", "change sample start", "change sample", "check position", "rotate wheel", "sample change complete", "sample rod up", "sample rod down", "retract rod in", "retract rod out", "insert rod in", "insert rod out", "wheel GV open", "wheel GV close", "vent source", "pump source", "shutdown"]
          }
        }
      }
      frame 8 {
        n204 = Increment(x=w380) -> (x+1=w366:u32)
        n205 = shared-variable "SCA-cRIO\\Mod8\\Sample Rod Actuator"(TRUE ("Sample Rod Actuator")) -> (error out=w371:errorcluster)  [unwired: 1 in]
        n206 = shared-variable ".\\local SCA shared var lib - old.lvlib\\Sample Rod Max Count"() -> (w364:u32)  [unwired: 1 in, 1 out]
        n207 = call "Modify array of SCA states.vi"("Current State"=w373, "Array of states to process"=w374) -> ("Next State"=w375:T6)  [unwired: 7 in, 1 out]
        n208 = shared-variable "SCA-cRIO\\global SCA shared var lib.lvlib\\Sample Rod status"(error in=w371) -> (w370:T4)  [unwired: 1 out]
        n209 = Greater Or Equal?(x=w366, y=w364) -> (x >= y?=w379:bool)
        n210 = shared-variable ".\\local SCA shared var lib - old.lvlib\\Sample Rod Min Count"() -> (w365:u32)  [unwired: 1 in, 1 out]
        n211 = Equal?(x=w370, y=Vertical_Rod_states."rod down") -> (x = y?=w368:bool)
        n212 = Select(t=w387, s=w368, f=u32 0) -> (s? t:f=w385:u32)
        n213 = Increment(x=w385) -> (x+1=w367:u32)
        n214 = Greater Or Equal?(x=w367, y=w365) -> (x >= y?=w386:bool)
        n215 = Select(t=w375, s=w386, f=w373) -> (s? t:f=w382:u16)
        n216 = case shown="True" w379 {
          tunnel: [w393 u32 0] -> w378
          tunnel: [w391 w394] -> w376
          tunnel: [w392 SCA_states."wait" ("SC2 state")] -> w381
          tunnel: w366 -> [w393 _]
          tunnel: w373 -> [w389 _]
          tunnel: [w388 "sample rod failure"] -> w383
          tunnel: w382 -> [w392 _]
          tunnel: w374 -> [w391 _]
          frame False {
            n217 = Format Into String(format string="%s", w389) -> (resulting string=w388:string)  [unwired: 2 in, 1 out]
          }
          frame True {
            w394 = T6[] [enum."wait", enum."insert rod out", enum."wait"] items=["initialize", "wait", "change sample start", "change sample", "check position", "rotate wheel", "sample change complete", "sample rod up", "sample rod down", "retract rod in", "retract rod out", "insert rod in", "insert rod out", "wheel GV open", "wheel GV close", "vent source", "pump source", "shutdown"]
          }
        }
      }
      frame 9 {
        n218 = Increment(x=w414) -> (x+1=w401:u32)
        n219 = shared-variable "SCA-cRIO\\Mod8\\Retract Rod Actuator"(TRUE ("Sample Rod Actuator")) -> (error out=w405:errorcluster)  [unwired: 1 in]
        n220 = shared-variable ".\\local SCA shared var lib - old.lvlib\\Retract Rod Max Count"() -> (w399:u32)  [unwired: 1 in, 1 out]
        n221 = call "Modify array of SCA states.vi"("Current State"=w407, "Array of states to process"=w408) -> ("Next State"=w409:T6)  [unwired: 7 in, 1 out]
        n222 = shared-variable "SCA-cRIO\\global SCA shared var lib.lvlib\\Retract Rod Status"(error in=w405) -> (w404:T3)  [unwired: 1 out]
        n223 = Greater Or Equal?(x=w401, y=w399) -> (x >= y?=w413:bool)
        n224 = shared-variable ".\\local SCA shared var lib - old.lvlib\\Retract Rod Min Count"() -> (w398:u32)  [unwired: 1 in, 1 out]
        n225 = Equal?(x=w404, y=Horizontal_Rod_states."rod in" ("Enum")) -> (x = y?=w403:bool)
        n226 = Select(t=w421, s=w403, f=u32 0) -> (s? t:f=w419:u32)
        n227 = Increment(x=w419) -> (x+1=w402:u32)
        n228 = Greater Or Equal?(x=w402, y=w398) -> (x >= y?=w420:bool)
        n229 = Select(t=w409, s=w420, f=w407) -> (s? t:f=w416:u16)
        n230 = case shown="True" w413 {
          tunnel: [w427 u32 0] -> w412
          tunnel: [w425 w428] -> w410
          tunnel: [w426 SCA_states."retract rod out" ("SC2 state")] -> w415
          tunnel: w401 -> [w427 _]
          tunnel: w407 -> [w423 _]
          tunnel: [w422 "retract rod failure"] -> w417
          tunnel: w416 -> [w426 _]
          tunnel: w408 -> [w425 _]
          frame False {
            n231 = Format Into String(format string="%s", w423) -> (resulting string=w422:string)  [unwired: 2 in, 1 out]
          }
          frame True {
            w428 = T6[] [enum."retract rod out", enum."insert rod out", enum."wait"] items=["initialize", "wait", "change sample start", "change sample", "check position", "rotate wheel", "sample change complete", "sample rod up", "sample rod down", "retract rod in", "retract rod out", "insert rod in", "insert rod out", "wheel GV open", "wheel GV close", "vent source", "pump source", "shutdown"]
          }
        }
      }
      frame 10 {
        n232 = Increment(x=w448) -> (x+1=w435:u32)
        n233 = shared-variable "SCA-cRIO\\Mod8\\Retract Rod Actuator"(FALSE ("Sample Rod Actuator")) -> (error out=w439:errorcluster)  [unwired: 1 in]
        n234 = call "Modify array of SCA states.vi"("Current State"=w441, "Array of states to process"=w442) -> ("Next State"=w443:T6)  [unwired: 7 in, 1 out]
        n235 = shared-variable ".\\local SCA shared var lib - old.lvlib\\Retract Rod Max Count"() -> (w433:u32)  [unwired: 1 in, 1 out]
        n236 = shared-variable "SCA-cRIO\\global SCA shared var lib.lvlib\\Retract Rod Status"(error in=w439) -> (w438:T3)  [unwired: 1 out]
        n237 = Greater Or Equal?(x=w435, y=w433) -> (x >= y?=w447:bool)
        n238 = shared-variable ".\\local SCA shared var lib - old.lvlib\\Retract Rod Min Count"() -> (w432:u32)  [unwired: 1 in, 1 out]
        n239 = Equal?(x=w438, y=Horizontal_Rod_states."rod out" ("Enum")) -> (x = y?=w437:bool)
        n240 = Select(t=w455, s=w437, f=u32 0) -> (s? t:f=w453:u32)
        n241 = Increment(x=w453) -> (x+1=w436:u32)
        n242 = Greater Or Equal?(x=w436, y=w432) -> (x >= y?=w454:bool)
        n243 = Select(t=w443, s=w454, f=w441) -> (s? t:f=w450:u16)
        n244 = case shown="False" w447 {
          tunnel: [w461 u32 0] -> w446
          tunnel: [w459 w462] -> w444
          tunnel: [w460 SCA_states."retract rod out" ("SC2 state")] -> w449
          tunnel: w435 -> [w461 _]
          tunnel: w441 -> [w457 _]
          tunnel: [w456 "retract rod failure"] -> w451
          tunnel: w450 -> [w460 _]
          tunnel: w442 -> [w459 _]
          frame False {
            n245 = Format Into String(format string="%s", w457) -> (resulting string=w456:string)  [unwired: 2 in, 1 out]
          }
          frame True {
            w462 = T6[] [enum."retract rod out", enum."insert rod out", enum."wait"] items=["initialize", "wait", "change sample start", "change sample", "check position", "rotate wheel", "sample change complete", "sample rod up", "sample rod down", "retract rod in", "retract rod out", "insert rod in", "insert rod out", "wheel GV open", "wheel GV close", "vent source", "pump source", "shutdown"]
          }
        }
      }
      frame 11 {
        n246 = Increment(x=w482) -> (x+1=w469:u32)
        n247 = shared-variable "SCA-cRIO\\Mod8\\Insert Rod Actuator"(TRUE ("Sample Rod Actuator")) -> (error out=w473:errorcluster)  [unwired: 1 in]
        n248 = call "Modify array of SCA states.vi"("Current State"=w475, "Array of states to process"=w476) -> ("Next State"=w477:T6)  [unwired: 7 in, 1 out]
        n249 = shared-variable ".\\local SCA shared var lib - old.lvlib\\Insert Rod Max Count"() -> (w467:u32)  [unwired: 1 in, 1 out]
        n250 = shared-variable "SCA-cRIO\\global SCA shared var lib.lvlib\\Insert Rod Status"(error in=w473) -> (w472:T3)  [unwired: 1 out]
        n251 = Greater Or Equal?(x=w469, y=w467) -> (x >= y?=w481:bool)
        n252 = shared-variable ".\\local SCA shared var lib - old.lvlib\\Insert Rod Min Count"() -> (w466:u32)  [unwired: 1 in, 1 out]
        n253 = Equal?(x=w472, y=Horizontal_Rod_states."rod in" ("Enum")) -> (x = y?=w471:bool)
        n254 = Select(t=w489, s=w471, f=u32 0) -> (s? t:f=w487:u32)
        n255 = Increment(x=w487) -> (x+1=w470:u32)
        n256 = Greater Or Equal?(x=w470, y=w466) -> (x >= y?=w488:bool)
        n257 = Select(t=w477, s=w488, f=w475) -> (s? t:f=w484:u16)
        n258 = case shown="True" w481 {
          tunnel: [w495 u32 0] -> w480
          tunnel: [w493 w496] -> w478
          tunnel: [w494 SCA_states."insert rod out" ("SC2 state")] -> w483
          tunnel: w469 -> [w495 _]
          tunnel: w475 -> [w491 _]
          tunnel: [w490 "insert rod failure"] -> w485
          tunnel: w484 -> [w494 _]
          tunnel: w476 -> [w493 _]
          frame False {
            n259 = Format Into String(format string="%s", w491) -> (resulting string=w490:string)  [unwired: 2 in, 1 out]
          }
          frame True {
            w496 = T6[] [enum."insert rod out", enum."retract rod out", enum."wait"] items=["initialize", "wait", "change sample start", "change sample", "check position", "rotate wheel", "sample change complete", "sample rod up", "sample rod down", "retract rod in", "retract rod out", "insert rod in", "insert rod out", "wheel GV open", "wheel GV close", "vent source", "pump source", "shutdown"]
          }
        }
      }
      frame 12 {
        n260 = Increment(x=w516) -> (x+1=w503:u32)
        n261 = shared-variable ".\\local SCA shared var lib - old.lvlib\\Insert Rod Max Count"() -> (w501:u32)  [unwired: 1 in, 1 out]
        n262 = shared-variable "SCA-cRIO\\Mod8\\Insert Rod Actuator"(FALSE ("Sample Rod Actuator")) -> (error out=w507:errorcluster)  [unwired: 1 in]
        n263 = call "Modify array of SCA states.vi"("Current State"=w509, "Array of states to process"=w510) -> ("Next State"=w511:T6)  [unwired: 7 in, 1 out]
        n264 = shared-variable "SCA-cRIO\\global SCA shared var lib.lvlib\\Insert Rod Status"(error in=w507) -> (w506:T3)  [unwired: 1 out]
        n265 = Greater Or Equal?(x=w503, y=w501) -> (x >= y?=w515:bool)
        n266 = shared-variable ".\\local SCA shared var lib - old.lvlib\\Insert Rod Min Count"() -> (w500:u32)  [unwired: 1 in, 1 out]
        n267 = Equal?(x=w506, y=Horizontal_Rod_states."rod out" ("Enum")) -> (x = y?=w505:bool)
        n268 = Select(t=w523, s=w505, f=u32 0) -> (s? t:f=w521:u32)
        n269 = Increment(x=w521) -> (x+1=w504:u32)
        n270 = Greater Or Equal?(x=w504, y=w500) -> (x >= y?=w522:bool)
        n271 = Select(t=w511, s=w522, f=w509) -> (s? t:f=w518:u16)
        n272 = case shown="False" w515 {
          tunnel: [w529 u32 0] -> w514
          tunnel: [w527 w530] -> w512
          tunnel: [w528 SCA_states."insert rod out" ("SC2 state")] -> w517
          tunnel: w503 -> [w529 _]
          tunnel: w509 -> [w525 _]
          tunnel: [w524 "insert rod failure"] -> w519
          tunnel: w518 -> [w528 _]
          tunnel: w510 -> [w527 _]
          frame False {
            n273 = Format Into String(format string="%s", w525) -> (resulting string=w524:string)  [unwired: 2 in, 1 out]
          }
          frame True {
            w530 = T6[] [enum."insert rod out", enum."retract rod out", enum."wait"] items=["initialize", "wait", "change sample start", "change sample", "check position", "rotate wheel", "sample change complete", "sample rod up", "sample rod down", "retract rod in", "retract rod out", "insert rod in", "insert rod out", "wheel GV open", "wheel GV close", "vent source", "pump source", "shutdown"]
          }
        }
      }
      frame 5 {
        w559 = 10000.0 ("acceleration")
        # "in motor steps"
        # "The counter logic here (along with \"wait position\") doesn't appear to have a clear purpose.  Doesn't appear that the failure state could ever be acheived as the max timer"
        n274 = shared-variable "SCA-cRIO\\global SCA shared var lib.lvlib\\New Move"() -> (w542:dbl)  [unwired: 1 in, 1 out]
        n275 = Increment(x=w556) -> (x+1=w551:u32)
        n276 = Increment(x=w558) -> (x+1=w541:u32)
        n277 = shared-variable ".\\local SCA shared var lib.lvlib\\Motor Status"(FALSE ("Motor Status")) -> ()  [unwired: 1 in, 1 out]
        n278 = feedback #1() -> (w536:bool)  [unwired: 1 in]
        n279 = xnode "Straight-Line Move"("resource"=w560, "execute"=w536, "position"=w542, "velocity"=w559, "acceleration"=w559, "deceleration"=w559, "accel. jerk"=w559, "smoothing"=w559) -> ("error out"=w539:errorcluster, "done"=w547:bool)  [unwired: 2 in, 4 out]
        "done" <- w547
        "Rotate Wheel error" <- w539
        n280 = shared-variable ".\\local SCA shared var lib - old.lvlib\\Rotate Wheel Min Count"() -> (w535:u32)  [unwired: 1 in, 1 out]
        n281 = shared-variable ".\\local SCA shared var lib.lvlib\\Rotate Wheel error"(w539) -> ()  [unwired: 1 in, 1 out]
        n282 = Not(x=w547) -> (.not. x?=w537:bool)
        n283 = feedback-in #1(w537) -> ()
        n284 = local write "Execute Move"(w537) -> ()
        n285 = shared-variable ".\\local SCA shared var lib - old.lvlib\\Rotate Wheel Max Count"() -> (w534:u32)  [unwired: 1 in, 1 out]
        n286 = Greater Or Equal?(x=w541, y=w535) -> (x >= y?=w552:bool)
        n287 = Select(t=u32 0, s=w552, f=w551) -> (s? t:f=w549:u32)
        n288 = Select(t=SCA_states."wait position" ("SC2 state"), s=w547, f=SCA_states."rotate wheel" ("SC2 state")) -> (s? t:f=w548:u16)
        n289 = Greater Or Equal?(x=w551, y=w534) -> (x >= y?=w557:bool)
        n290 = case shown="False" w557 {
          tunnel: [w561 w566] -> w555
          tunnel: [w565 SCA_states."retract rod out" ("SC2 state")] -> w554
          tunnel: w545 -> [w563 _]
          tunnel: [w562 "rotate failure"] -> w553
          tunnel: w548 -> [w565 _]
          tunnel: w546 -> [w561 _]
          frame False {
            n291 = Format Into String(format string="%s", w563) -> (resulting string=w562:string)  [unwired: 2 in, 1 out]
          }
          frame True {
            w566 = T6[] [enum."retract rod out", enum."insert rod out", enum."wait"] items=["initialize", "wait", "change sample start", "change sample", "check position", "rotate wheel", "sample change complete", "sample rod up", "sample rod down", "retract rod in", "retract rod out", "insert rod in", "insert rod out", "wheel GV open", "wheel GV close", "vent source", "pump source", "shutdown"]
          }
        }
      }
      frame 5 {
        # "It's still unclear the purpose of \"wait posiiton\" state given the logic withi -- . could probably be replaced by having timing check in \"check position\" state (similar to what is done in the SCB project's state machine"
        n292 = Increment(x=w611) -> (x+1=w612:u32)
        n293 = Increment(x=w609) -> (x+1=w605:u32)
        n294 = shared-variable ".\\local SCA shared var lib - old.lvlib\\Wait Position Min Count"() -> (w595:u32)  [unwired: 1 in, 1 out]
        n295 = shared-variable ".\\local SCA shared var lib - old.lvlib\\Wait Position Max Count"() -> (w610:u32)  [unwired: 1 in, 1 out]
        n296 = Greater Or Equal?(x=w612, y=w595) -> (x >= y?=w606:bool)
        n297 = Greater Or Equal?(x=w605, y=w610) -> (x >= y?=w602:bool)
        n298 = Select(t=u32 0, s=w606, f=w605) -> (s? t:f=w603:u32)
        n299 = case shown="True" w602 {
          tunnel: [w616 w617] -> w608
          tunnel: w600 -> [w614 _]
          tunnel: [w613 "rotate failure"] -> w607
          tunnel: w599 -> [w616 _]
          frame False {
            n300 = Format Into String(format string="%s", w614) -> (resulting string=w613:string)  [unwired: 2 in, 1 out]
          }
          frame True {
            w617 = T6[] [enum."retract rod out", enum."insert rod out", enum."wait"] items=["initialize", "wait", "change sample start", "change sample", "check position", "rotate wheel", "sample change complete", "sample rod up", "sample rod down", "retract rod in", "retract rod out", "insert rod in", "insert rod out", "wheel GV open", "wheel GV close", "vent source", "pump source", "shutdown"]
          }
        }
        n301 = Select(t=SCA_states."wait position" ("SC2 state"), s=w602, f=SCA_states."check position" ("SC2 state")) -> (s? t:f=w601:u16)
      }
      frame 4 {
        # "Move in motor steps"
        n302 = shared-variable "SCA-cRIO\\global SCA shared var lib.lvlib\\Encoder position"() -> (w624:i16)  [unwired: 1 in, 1 out]
        n303 = shared-variable ".\\local SCA shared var lib.lvlib\\Encoder Offset"() -> (w625:i16)  [unwired: 1 in, 1 out]
        n304 = shared-variable ".\\global SCA shared var lib.lvlib\\New sample"() -> (w621:i8)  [unwired: 1 in, 1 out]
        n305 = call "SCA Sample-Encoder conversion.vi"("Step Window Radius"="Step Window Radius", "Rollover Sample"="Rollover Sample", "Encoder Offset"=w624, "Encoder Position"=w625, "Desired Sample"=w621) -> ("Window limit 1"=w620:i16, "Within Range?"=w633:bool, "Encoder destination"=w631:i16, "Window limit 2"=w619:i16, "New move (encoder steps)"=w636:i16)  [unwired: 2 in]
        "Encoder Destination" <- w631
        "In Range?" <- w633
        "Window Limit 2" <- w619
        "Window Limit 1" <- w620
        n306 = shared-variable "SCA-cRIO\\old - shared var lib.lvlib\\wheel offset plus"(w620) -> ()  [unwired: 1 in, 1 out]
        n307 = shared-variable "SCA-cRIO\\global SCA shared var lib.lvlib\\Encoder Destination"(w631) -> ()  [unwired: 1 in, 1 out]
        n308 = shared-variable "SCA-cRIO\\old - shared var lib.lvlib\\wheel offset minus"(w619) -> ()  [unwired: 1 in, 1 out]
        n309 = call "Modify array of SCA states.vi"("Current State"=w630, "Array of states to process"=w629) -> ("Next State"=w628:T6)  [unwired: 7 in, 1 out]
        n310 = Select(t=w628, s=w633, f=SCA_states."rotate wheel" ("SC2 state")) -> (s? t:f=w640:T6)
        n311 = shared-variable ".\\local SCA shared var lib.lvlib\\Motor Status"(w633) -> ()  [unwired: 1 in, 1 out]
        n312 = Multiply(x=w636, y=3.0519) -> (x*y=w632:dbl)
        "New Move" <- w632
        n313 = shared-variable "SCA-cRIO\\global SCA shared var lib.lvlib\\New Move"(w632) -> ()  [unwired: 1 in, 1 out]
        n314 = Format Into String(format string="%s", w630) -> (resulting string=w639:string)  [unwired: 2 in, 1 out]
      }
    }
    "action" <- w219
    "SCA next state" <- w223
    n315 = shared-variable "SCA-cRIO\\global SCA shared var lib.lvlib\\Current State"(w213) -> ()  [unwired: 1 in, 1 out]
    n316 = call "Wait Until Next Multiple"("Count(mSec)"=u32 5) -> ()  [unwired: 1 out]
    n317 = shared-variable "SCA-cRIO\\global SCA shared var lib.lvlib\\SC SM counter"(w215) -> ()  [unwired: 1 in, 1 out]
  }
  n318 = while {
    tunnel: w9 -> [w646]
    stop <- FALSE ("stop 3") stop-if-true
    # "Convectron readback - GP375 Convectron uses thermocouple gauge to measure pressure on wheel chamber"
    n319 = Concatenate Strings("RD" ("write buffer 2"), "\r") -> (w653:string)
    n320 = Wait Until Next ms Multiple(millisecond multiple=u32 2000) -> ()  [unwired: 1 out]
    n321 = VISA Write(VISA resource name=w646, write buffer=w653) -> (VISA resource name out=w647:refnum<visa-resource-name>, error out=w643:errorcluster)  [unwired: 1 in, 1 out]
    n322 = property class="Instr"(reference=w647, error in=w643) -> (reference out=w648:refnum<visa-resource-name>, error out=w642:errorcluster, "Bytes at Port"=w649:u32)
    n323 = VISA Read(VISA resource name=w648, byte count=w649, error in (no error)=w642) -> (read buffer=w644:string, error out=w641:errorcluster)  [unwired: 2 out]
    "Sample Wheel Convectron" <- w644
    "Convectron readback loop error" <- w641
    n324 = shared-variable ".\\local SCA shared var lib.lvlib\\Convectron readback loop error"(w641) -> ()  [unwired: 1 in, 1 out]
    n325 = shared-variable "SCA-cRIO\\global SCA shared var lib.lvlib\\Sample Wheel Convectron"(w644) -> ()  [unwired: 1 in, 1 out]
  }
  n326 = while {
    tunnel: w14 -> [w657]
    tunnel: w20 -> [w660]
    stop <- FALSE ("stop 4") stop-if-true
    w656 = 3.0 ("Delay Time (s)")
    # "GP307 readback for both controllers on SCA - Bellows readings in and around sample rods upper position; Ion source readings are in and around source region"
    n327 = Wait Until Next ms Multiple(millisecond multiple=u32 500) -> ()  [unwired: 1 out]
    n328 = call "GP307 Read-RT.vi"("Delay Time (s)"=w656, "VISA Refnum in"=w660) -> ("error out"=w658:errorcluster, "GP307 output"=w659:T2)  [unwired: 7 in, 1 out]
    "Bellows Vac Cluster" <- w659
    n329 = call "GP307 Read-RT.vi"("Delay Time (s)"=w656, "VISA Refnum in"=w657) -> ("error out"=w654:errorcluster, "GP307 output"=w655:T2)  [unwired: 7 in, 1 out]
    "Ion Source Vac Cluster" <- w655
    n330 = shared-variable "SCA-cRIO\\global SCA shared var lib.lvlib\\Bellows Vac Cluster"(w659) -> ()  [unwired: 1 in, 1 out]
    n331 = shared-variable "SCA-cRIO\\global SCA shared var lib.lvlib\\Ion Source Vac Cluster"(w655) -> ()  [unwired: 1 in, 1 out]
    n332 = Merge Errors(w658, w654) -> (w661:errorcluster)
    "Vac Readback Loop error" <- w661
    n333 = shared-variable ".\\local SCA shared var lib.lvlib\\Vac Readback Loop error"(w661) -> ()  [unwired: 1 in, 1 out]
  }
  n334 = while {
    stop <- FALSE stop-if-true
    n335 = shared-variable "SCA-cRIO\\legacy SCA shared var.lvlib\\Pump out Source"() -> (w665:bool)  [unwired: 1 in, 1 out]
    "Pumping out Source" <- w665
    n336 = Wait Until Next ms Multiple(millisecond multiple=u32 100) -> ()  [unwired: 1 out]
    n337 = case shown="True" w665 {
      frame False {
      }
      frame True {
        n338 = shared-variable "SCA-cRIO\\legacy SCA shared var.lvlib\\Pump out Source"(FALSE ("rod up shared")) -> ()  [unwired: 1 in, 1 out]
        n339 = shared-variable ".\\local SCA shared var lib.lvlib\\SCA state control"(SCA_states."pump source" ("SCA state control")) -> ()  [unwired: 1 in, 1 out]
      }
    }
  }
  n340 = while {
    stop <- FALSE stop-if-true
    n341 = shared-variable "SCA-cRIO\\legacy SCA shared var.lvlib\\Close Wheel GV"() -> (w669:bool)  [unwired: 1 in, 1 out]
    "Close Wheel GV" <- w669
    n342 = Wait Until Next ms Multiple(millisecond multiple=u32 50) -> ()  [unwired: 1 out]
    n343 = case shown="True" w669 {
      frame False {
      }
      frame True {
        n344 = shared-variable "SCA-cRIO\\legacy SCA shared var.lvlib\\Close Wheel GV"(FALSE ("rod up shared")) -> ()  [unwired: 1 in, 1 out]
        n345 = shared-variable ".\\local SCA shared var lib.lvlib\\SCA state control"(SCA_states."wheel GV close" ("SC2 state")) -> ()  [unwired: 1 in, 1 out]
      }
    }
  }
  n346 = while {
    stop <- FALSE ("stop") stop-if-true
    n347 = shared-variable "SCA-cRIO\\Mod7\\Wheel GV OPEN sensor"() -> (w697:bool, error out=w683:errorcluster)  [unwired: 1 in]
    n348 = shared-variable "SCA-cRIO\\Mod7\\Wheel GV CLOSED sensor"(error in=w683) -> (w698:bool, error out=w682:errorcluster)
    n349 = Wait Until Next ms Multiple(millisecond multiple=u32 50) -> ()  [unwired: 1 out]
    n350 = shared-variable "SCA-cRIO\\Mod7\\Retract Rod IN sensor"() -> (w692:bool, error out=w685:errorcluster)  [unwired: 1 in]
    "Retract Rod IN sensor" <- w692
    n351 = shared-variable "SCA-cRIO\\Mod7\\Retract Rod OUT sensor"(error in=w685) -> (w691:bool, error out=w679:errorcluster)
    "Retract Rod OUT sensor" <- w691
    n352 = shared-variable "SCA-cRIO\\Mod7\\Insert Rod IN sensor"() -> (w690:bool, error out=w684:errorcluster)  [unwired: 1 in]
    "Insert Rod IN sensor" <- w690
    n353 = shared-variable "SCA-cRIO\\Mod7\\Insert Rod OUT sensor"(error in=w684) -> (w689:bool, error out=w681:errorcluster)
    "Insert Rod OUT sensor" <- w689
    n354 = shared-variable "SCA-cRIO\\Mod7\\Sample Rod UP sensor"() -> (w695:bool, error out=w686:errorcluster)  [unwired: 1 in]
    "Sample Rod UP sensor" <- w695
    n355 = shared-variable "SCA-cRIO\\Mod7\\Sample Rod DOWN sensor"(error in=w686) -> (w694:bool, error out=w680:errorcluster)
    "Sample Rod DOWN sensor" <- w694
    n356 = Bundle By Name(cluster=T5 {"OPEN sensor"=FALSE, "Closed sensor"=FALSE} ("Gate Valve"), "OPEN sensor"=w697, "Closed sensor"=w698) -> (w700:T5)
    "Wheel GV" <- w700
    n357 = call "Horizontal Rod Sensor-State converter.vi"("IN Sensor"=w690, "OUT Sensor"=w689) -> ("Status"=w688:T3)  [unwired: 8 in]
    "Insert Rod Status" <- w688
    n358 = call "Horizontal Rod Sensor-State converter.vi"("IN Sensor"=w692, "OUT Sensor"=w691) -> ("Status"=w687:T3)  [unwired: 8 in]
    "Retract Rod Status" <- w687
    n359 = call "Vertical Rod Sensor-State converter.vi"("UP Sensor"=w695, "DOWN Sensor"=w694) -> ("Status"=w693:T4)  [unwired: 8 in]
    "Sample Rod status" <- w693
    n360 = shared-variable "SCA-cRIO\\global SCA shared var lib.lvlib\\Retract Rod Status"(w687, error in=w679) -> (error out=w676:errorcluster)
    n361 = shared-variable "SCA-cRIO\\global SCA shared var lib.lvlib\\Insert Rod Status"(w688, error in=w681) -> (error out=w675:errorcluster)
    n362 = call "GV status converter.vi"("Gate Valve"=w700) -> ("GV Status"=w696:T9)  [unwired: 10 in]
    n363 = shared-variable "SCA-cRIO\\global SCA shared var lib.lvlib\\Sample Rod status"(w693, error in=w680) -> (error out=w677:errorcluster)
    n364 = shared-variable "SCA-cRIO\\global SCA shared var lib.lvlib\\Wheel GV Status"(w696, error in=w682) -> (error out=w674:errorcluster)
    n365 = Merge Errors(w677, w676, w675, w674) -> (w678:errorcluster)
    "Sensor loop error" <- w678
    n366 = shared-variable ".\\local SCA shared var lib.lvlib\\Sensor Loop error"(w678) -> ()  [unwired: 1 in, 1 out]
  }
  n367 = node-c288() -> (w5:T10)  [unwired: 4 in]
  n368 = timed-loop {
    timing: w5 -> [_]
    timing-out: [_] -> w4
    stop <- FALSE stop-if-true
    # "Encoder readback loop"
    n369 = node-c288() -> ()  [unwired: 1 in, 1 out]
    n370 = shared-variable "SCA-cRIO\\Mod6\\DIO0"() -> (w735:bool, error out=w718:errorcluster)  [unwired: 1 in]
    n371 = shared-variable "SCA-cRIO\\Mod6\\DIO1"(error in=w718) -> (w734:bool, error out=w717:errorcluster)
    n372 = shared-variable "SCA-cRIO\\Mod6\\DIO2"(error in=w717) -> (w725:bool, error out=w716:errorcluster)
    n373 = shared-variable "SCA-cRIO\\Mod6\\DIO3"(error in=w716) -> (w724:bool, error out=w715:errorcluster)
    n374 = shared-variable "SCA-cRIO\\Mod6\\DIO4"(error in=w715) -> (w733:bool, error out=w714:errorcluster)
    n375 = shared-variable "SCA-cRIO\\Mod6\\DIO5"(error in=w714) -> (w732:bool, error out=w713:errorcluster)
    n376 = shared-variable "SCA-cRIO\\Mod6\\DIO6"(error in=w713) -> (w731:bool, error out=w712:errorcluster)
    n377 = shared-variable "SCA-cRIO\\Mod6\\DIO7"(error in=w712) -> (w711:bool, error out=w710:errorcluster)
    n378 = shared-variable "SCA-cRIO\\Mod6\\DIO8"(error in=w710) -> (w730:bool, error out=w709:errorcluster)
    n379 = shared-variable "SCA-cRIO\\Mod6\\DIO9"(error in=w709) -> (w723:bool, error out=w708:errorcluster)
    n380 = shared-variable "SCA-cRIO\\Mod6\\DIO10"(error in=w708) -> (w729:bool, error out=w707:errorcluster)
    n381 = shared-variable "SCA-cRIO\\Mod6\\DIO11"(error in=w707) -> (w728:bool, error out=w706:errorcluster)
    n382 = shared-variable "SCA-cRIO\\Mod6\\DIO12"(error in=w706) -> (w727:bool, error out=w705:errorcluster)
    n383 = shared-variable "SCA-cRIO\\Mod6\\DIO13"(error in=w705) -> (w726:bool, error out=w704:errorcluster)
    n384 = Bundle By Name(cluster=T13 {"MSB"=FALSE, "13th bit"=FALSE, "12th bit"=FALSE, "11th bit"=FALSE, "10th bit"=FALSE, "9th bit"=FALSE, "8th bit"=FALSE, "7th bit"=FALSE, "6th bit"=FALSE, "5th bit"=FALSE, "4th bit"=FALSE, "3rd bit"=FALSE, "2nd bit"=FALSE, "LSB"=FALSE} ("Cluster"), "MSB"=w735, "13th bit"=w734, "12th bit"=w725, "11th bit"=w724, "10th bit"=w733, "9th bit"=w732, "8th bit"=w731, "7th bit"=w711, "6th bit"=w730, "5th bit"=w723, "4th bit"=w729, "3rd bit"=w728, "2nd bit"=w727, "LSB"=w726) -> (w737:T13)
    n385 = call "Encoder-Decoder.vi"("Encoder data"=w737) -> ("Raw bits"=→"Raw bits":bool[], "Converted bits"=→"Converted bits":bool[], "Encoder position"=w722:u16)  [unwired: 8 in]
    "Encoder position" <- w722
    n386 = shared-variable "SCA-cRIO\\global SCA shared var lib.lvlib\\Encoder position"(w722, error in=w704) -> (error out=w703:errorcluster)
    "Encoder loop error" <- w703
    n387 = shared-variable ".\\local SCA shared var lib.lvlib\\Encoder loop error"(w703) -> ()  [unwired: 1 in, 1 out]
    n388 = node-c288() -> ()  [unwired: 1 in, 1 out]
  }
  n389 = while {
    stop <- FALSE stop-if-true
    n390 = shared-variable "SCA-cRIO\\legacy SCA shared var.lvlib\\Sample Rod retraction"() -> (w741:bool)  [unwired: 1 in, 1 out]
    "retract Sample Rod" <- w741
    n391 = Wait Until Next ms Multiple(millisecond multiple=u32 100) -> ()  [unwired: 1 out]
    n392 = case shown="True" w741 {
      frame False {
      }
      frame True {
        n393 = shared-variable "SCA-cRIO\\legacy SCA shared var.lvlib\\Sample Rod retraction"(FALSE ("rod up shared")) -> ()  [unwired: 1 in, 1 out]
        n394 = shared-variable ".\\local SCA shared var lib.lvlib\\SCA state control"(SCA_states."sample rod up" ("SCA state control")) -> ()  [unwired: 1 in, 1 out]
      }
    }
  }
  n395 = while {
    stop <- FALSE stop-if-true
    n396 = shared-variable "SCA-cRIO\\legacy SCA shared var.lvlib\\Insert Rod retraction"() -> (w746:bool)  [unwired: 1 in, 1 out]
    "retract Insert Rod" <- w746
    n397 = Wait Until Next ms Multiple(millisecond multiple=u32 100) -> ()  [unwired: 1 out]
    n398 = case shown="True" w746 {
      frame False {
      }
      frame True {
        n399 = shared-variable "SCA-cRIO\\legacy SCA shared var.lvlib\\Insert Rod retraction"(FALSE ("rod up shared")) -> ()  [unwired: 1 in, 1 out]
        n400 = shared-variable ".\\local SCA shared var lib.lvlib\\SCA state control"(SCA_states."insert rod out" ("SC2 state")) -> ()  [unwired: 1 in, 1 out]
      }
    }
  }
  n401 = while {
    stop <- FALSE stop-if-true
    n402 = shared-variable "SCA-cRIO\\legacy SCA shared var.lvlib\\Retract Rod retraction"() -> (w751:bool)  [unwired: 1 in, 1 out]
    "retract Retract Rod" <- w751
    n403 = Wait Until Next ms Multiple(millisecond multiple=u32 100) -> ()  [unwired: 1 out]
    n404 = case shown="True" w751 {
      frame False {
      }
      frame True {
        n405 = shared-variable "SCA-cRIO\\legacy SCA shared var.lvlib\\Retract Rod retraction"(FALSE ("rod up shared")) -> ()  [unwired: 1 in, 1 out]
        n406 = shared-variable ".\\local SCA shared var lib.lvlib\\SCA state control"(SCA_states."retract rod out" ("SC2 state")) -> ()  [unwired: 1 in, 1 out]
      }
    }
  }
  n407 = while {
    stop <- FALSE stop-if-true
    n408 = shared-variable "SCA-cRIO\\legacy SCA shared var.lvlib\\Retract Rod insertion"() -> (w756:bool)  [unwired: 1 in, 1 out]
    "insert Retract Rod" <- w756
    n409 = Wait Until Next ms Multiple(millisecond multiple=u32 100) -> ()  [unwired: 1 out]
    n410 = case shown="True" w756 {
      frame False {
      }
      frame True {
        n411 = shared-variable "SCA-cRIO\\legacy SCA shared var.lvlib\\Retract Rod insertion"(FALSE ("rod up shared")) -> ()  [unwired: 1 in, 1 out]
        n412 = shared-variable ".\\local SCA shared var lib.lvlib\\SCA state control"(SCA_states."retract rod in" ("SC2 state")) -> ()  [unwired: 1 in, 1 out]
      }
    }
  }
  n413 = while {
    stop <- FALSE stop-if-true
    n414 = shared-variable "SCA-cRIO\\legacy SCA shared var.lvlib\\Sample Rod insertion"() -> (w761:bool)  [unwired: 1 in, 1 out]
    "insert Sample Rod" <- w761
    n415 = Wait Until Next ms Multiple(millisecond multiple=u32 100) -> ()  [unwired: 1 out]
    n416 = case shown="True" w761 {
      frame False {
      }
      frame True {
        n417 = shared-variable "SCA-cRIO\\legacy SCA shared var.lvlib\\Sample Rod insertion"(FALSE ("rod up shared")) -> ()  [unwired: 1 in, 1 out]
        n418 = shared-variable ".\\local SCA shared var lib.lvlib\\SCA state control"(SCA_states."sample rod down" ("SC2 state")) -> ()  [unwired: 1 in, 1 out]
      }
    }
  }
  n419 = while {
    stop <- FALSE stop-if-true
    n420 = shared-variable "SCA-cRIO\\legacy SCA shared var.lvlib\\Insert Rod insertion"() -> (w766:bool)  [unwired: 1 in, 1 out]
    "insert Insert Rod" <- w766
    n421 = Wait Until Next ms Multiple(millisecond multiple=u32 100) -> ()  [unwired: 1 out]
    n422 = case shown="True" w766 {
      frame False {
      }
      frame True {
        n423 = shared-variable "SCA-cRIO\\legacy SCA shared var.lvlib\\Insert Rod insertion"(FALSE ("rod up shared")) -> ()  [unwired: 1 in, 1 out]
        n424 = shared-variable ".\\local SCA shared var lib.lvlib\\SCA state control"(SCA_states."insert rod in" ("SC2 state")) -> ()  [unwired: 1 in, 1 out]
      }
    }
  }
  n425 = node-c288(w4) -> ()  [unwired: 1 out]
  n426 = disable-structure shown="Disabled" {
    frame Disabled {
      n427 = while {
        stop <- FALSE stop-if-true
        # "What is this now?"
        n428 = shared-variable "SCA-cRIO\\old - shared var lib.lvlib\\rezero"() -> (w771:bool)  [unwired: 1 in, 1 out]
        n429 = Wait Until Next ms Multiple(millisecond multiple=u32 100) -> ()  [unwired: 1 out]
        n430 = case shown="True" w771 {
          frame False {
          }
          frame True {
            n431 = shared-variable "SCA-cRIO\\old - shared var lib.lvlib\\rezero"(FALSE ("rod up shared")) -> ()  [unwired: 1 in, 1 out]
            n432 = shared-variable ".\\local SCA shared var lib.lvlib\\SCA state control"(SCA_states."initialize" ("SC2 state")) -> ()  [unwired: 1 in, 1 out]
          }
        }
      }
      n433 = local write item#-1(T14 "rezero" ("state control")) -> ()
    }
    frame Enabled {
    }
  }
  n434 = disable-structure shown="Disabled" {
    frame Disabled {
      # "Was in sensor/acutator loop"
      n435 = shared-variable "SCA-cRIO\\old - shared var lib.lvlib\\change sample start end"() -> (→"change sample start end":bool)  [unwired: 1 in, 1 out]
      n436 = shared-variable "SCA-cRIO\\old - shared var lib.lvlib\\start sample change"() -> (→"start sample change":bool)  [unwired: 1 in, 1 out]
    }
    frame Enabled {
    }
  }
  n437 = while {
    stop <- FALSE stop-if-true
    # "What is this now?"
    n438 = shared-variable "SCA-cRIO\\old - shared var lib.lvlib\\set encoder wheel"() -> (w778:bool)  [unwired: 1 in, 1 out]
    n439 = Wait Until Next ms Multiple(millisecond multiple=u32 100) -> ()  [unwired: 1 out]
    n440 = case shown="True" w778 {
      frame False {
      }
      frame True {
        n441 = shared-variable "SCA-cRIO\\old - shared var lib.lvlib\\set encoder wheel"(FALSE ("rod up shared")) -> ()  [unwired: 1 in, 1 out]
        n442 = shared-variable ".\\local SCA shared var lib.lvlib\\SCA state control"(SCA_states."initialize" ("SC2 state")) -> ()  [unwired: 1 in, 1 out]
      }
    }
  }
  n443 = while {
    stop <- FALSE stop-if-true
    n444 = Wait Until Next ms Multiple(millisecond multiple=u32 50) -> ()  [unwired: 1 out]
  }
  n445 = disable-structure shown="Disabled" {
    frame Disabled {
      (unwired) 2794.0 ("y")
      (unwired) 2730.0 ("y")
      (unwired) 2613.0 ("y")
      (unwired) u32 16838 ("x")
      # "had been in check position case"
    }
    frame Enabled {
    }
  }
